vi "MoD Main-Optimize - HPLCv2 HWE.vi"() -> ()   [LabVIEW 2015]
uses:
  <vilib>/silver_ctls/ArrayMatrixCluster/Real Matrix NI_Silver.ctl
  <vilib>/ni845x/ni845x.llb/ni845xControl.ctl
  <vilib>/MakerHub/LINX/Public/Peripherals/Analog/Analog Read 1 Chan.vi
  <vilib>/MakerHub/LINX/Public/Peripherals/Analog/Analog Read N Chans.vi
  <vilib>/MakerHub/LINX/Public/Peripherals/Digital/Digital Write 1 Chan.vi
  <vilib>/MakerHub/LINX/Private/Local IO/LinxAnalogRead.vi
  <vilib>/MakerHub/LINX/Public/Utilities/Check Channel.vi
  <vilib>/MakerHub/LINX/Public/Peripherals/Digital/Digital Write N Chans.vi
  <vilib>/MakerHub/LINX/Private/Local IO/LinxDigitalWrite.vi
  <vilib>/addons/control/pid/pid.llb/PID Control Input Filter (DBL).vi
  <vilib>/MakerHub/LINX/Private/Utilties/Generate Error.vi
  <vilib>/addons/control/pid/autopid.llb/PID Online Autotuning (Relay Feedback).vi
  <vilib>/Analysis/Matrix/Numeric/Conversions/Array To Matrix - RA2.vi
  <vilib>/ni845x/ni845x.llb/NI-845x Close Device Reference.vi
  <vilib>/addons/control/pid/NI_PID_autopid.lvlib
  <vilib>/addons/control/pid/NI_PID_pid.lvlib
  <vilib>/Analysis/Matrix/NI_Matrix.lvlib
  <vilib>/MakerHub/LINX/LMH-LINX.lvlib
  <instrlib>/Harvard Apparatus PHD Ultra Series/Harvard Apparatus PHD Ultra Series.lvlib
panel:
  out "running?":bool=TRUE
  out "new_reactor_volume":bool[](array[boolean])
  out "new_reactor_length":bool[](array[boolean])
  out "Phase_Sensor_voltage":dbl
  out "P_tot":dbl
  out "pause for ms":bool=TRUE
  out "stop_xl_write":bool=TRUE
  out "Num_exp_till_pause":i32
  out "Syringe_pump?":bool=TRUE
  out "System Error":bool=TRUE
  out "error out":errorcluster
  out "Pump setpoint(ul/min) 6":dbl format="%#_13g"
  out "Pump setpoint(ul/min) 5":dbl format="%#_13g"
  out "Pump setpoint(ul/min) 4":dbl format="%#_13g"
  out "Pump setpoint(ul/min) 3":dbl format="%#_13g"
  out "Pump setpoint(ul/min) 2":dbl format="%#_13g"
  out "Pump setpoint(ul/min) 1":dbl format="%#_13g"
  out "Volume (ul) 5":dbl format="%#_13g"
  out "Volume (ul) 4":dbl format="%#_13g"
  out "Volume (ul) 3":dbl format="%#_13g"
  out "Volume (ul) 2":dbl format="%#_13g"
  out "Volume (ul) 1":dbl format="%#_13g"
  in  "tau 5":dbl format="%#_13g"
  out "tau 4":dbl format="%#_13g"
  out "tau 3":dbl format="%#_13g"
  out "tau 2":dbl format="%#_13g"
  out "tau 1":dbl format="%#_13g"
  out "Reactor Length":dbl format="%#_13g"
  out "Flowrate Sensor 2":dbl format="%#_13g"
  out "Flowrate Sensor 1":dbl format="%#_13g"
  out "Pressure 2":dbl format="%#_13g"
  out "Pressure 1":dbl format="%#_13g"
  out "Temperature Control 5":bool=TRUE
  out "Temperature Control 4":bool=TRUE
  out "Temperature Control 3":bool=TRUE
  out "Temperature Control 2":bool=TRUE
  out "Temperature Control 1":bool=TRUE
  out "Temperature SP 5":dbl format="%#_g'C"
  out "Temperature SP 4":dbl format="%#_g'C"
  out "Temperature SP 3":dbl format="%#_g'C"
  out "Temperature SP 2":dbl format="%#_g'C"
  out "Temperature SP 1":dbl format="%#_g'C"
  in  "Bay Temperature 5":dbl
  in  "SSR Duration 5":dbl
  in  "SSR Duration 4":dbl
  in  "SSR Duration 3":dbl
  in  "SSR Duration 2":dbl
  in  "SSR Duration 1":dbl
  in  "Total Product Amount":dbl=1.0 format="%#_gml"
  out "Setup Error":bool=TRUE
  out "Error Message":string
  out "ID CTR":i32
  in  "Tab Control":T1(tab)
  out "Reagent pic 5":picture
  in  "reagent name 5":string
  out "Reagent Pic 4":picture
  in  "reagent name 4":string
  out "Reagent Pic 3":picture
  in  "reagent  name 3":string="4-phenylcyclohexanone"
  in  "Product name":string
  in  "reagent name 1":string="Triethyl phosphonoacetate"
  out "Reagent Pic 1":picture
  in  "Vr5":dbl format="%#_guL"
  in  "Vr4":dbl format="%#_guL"
  in  "Vr3":dbl format="%#_guL"
  in  "Vr2":dbl format="%#_guL"
  in  "Vr1":dbl format="%#_guL"
  in  "System decide help Button":bool
  in  "Reaction Scheme Confirm":bool
  in  "Synthesis Route Array":string[][](array[string])=[["Triethyl phosphonoacetate", "0.2", "PhB(OH)2", "", "", ""], ["potassium tert-butoxide", "0.5", "-", "-", "-", "-"], ["4-phenylcyclohexanone", "0.2", "-", "-", "-", "-"], ["", "", "-", "-", "-", "-"]]
  in  "System decide help Button 2":bool
  out "Setup Confirm":bool=TRUE
  in  "BAY 1":u16(ring)=2 items=["               Bypass", "         Heated Reactor", "    Small Heated Reator", "         Cooled Reactor", "      Packed Bed Reactor", "          Photo Reactor", "             Separator"]
  in  "BAY 5":u16(ring) items=["               Bypass", "         Heated Reactor", "    Small Heated Reactor", "         Cooled Reactor", "     Packed Bed Reactor", "         Photo Reactor", "             Separator"]
  in  "BAY 4":u16(ring) items=["                Bypass", "         Heated Reactor", "    Small Heated Reactor", "         Cooled Reactor", "     Packed Bed Reactor", "         Photo Reactor", "             Separator"]
  in  "BAY 3":u16(ring) items=["               Bypass", "         Heated Reactor", "    Small Heated Reactor", "         Cooled Reactor", "     Packed Bed Reactor", "          Photo Reactor", "             Separator"]
  in  "BAY 2":u16(ring)=1 items=["               Bypass", "         Heated Reactor", "    Small Heated Reactor", "         Cooled Reactor", "      Packed Bed Reactor", "          Photo Reactor", "             Separator"]
  out "Reagent Pic 2":picture
  out "Product Pic":picture
  in  "reagent name 2":string="potassium tert-butoxide"
  in  "reagent name 6":string
  out "Reagent Pic 6":picture
  in  "System Parameters Help Button":bool
  out "Setup Confirm 2":bool
  in  "System Parameters Confirm Button":bool
  in  "Bay Parameters":T2={"Bay 1 "={"Pump 1 Flowrate"=0.0, "optimize_temp"=TRUE, "optimize_tau"=TRUE, "Run at set flowrate"=FALSE, "Pump 2 Flowrate"=0.0, "Temperature Params"=[40.0, 100.0, 100.0], "pump params 1"=[22.6, 226.0, 325.0], "pump params 2"=[22.6, 226.0, 325.0], "Temperature"=0.0, "Run at set temperature"=FALSE}, "Bay 2 "={"Pump 3 Flowrate"=0.0, "optimize_temp"=TRUE, "optimize_tau"=FALSE, "Run at set flowrate"=TRUE, "Temperature Params"=[40.0, 100.0, 100.0], "Resisdence time params"=[40.6, 406.0, 650.0], "pump_at_ratio"=FALSE, "pump_num_ratio"=1.0, "Temperature"=0.0, "Run at set temperature"=FALSE}, "Bay 3 "={"Pump 4 Flowrate"=100.0, "optimize_temp"=FALSE, "optimize_tau"=FALSE, "Run at set flowrate"=FALSE, "Temperature Params"=[40.0, 100.0, 100.0], "Resisdence time params"=[47.0, 476.0, 0.0], "pump_at_ratio"=FALSE, "pump_num_ratio"=0.0, "Temperature "=0.0, "Run at set temperature"=FALSE}, "Bay 4 "={"Pump 5 Flowrate"=40.0, "Run at set flowrate"=FALSE, "optimize_temp"=FALSE, "optimize_tau"=TRUE, "Resisdence time params"=[40.6, 406.0, 225.0], "Temperature Params"=[40.0, 100.0, 80.0], "pump_at_ratio"=FALSE, "pump_num_ratio"=0.0, "Temperature"=0.0, "Run at set temperature"=FALSE}, "Bay 5 "={"Pump 6 Flowrate"=0.0, "Run at set flowrate"=FALSE, "optimize_temp"=FALSE, "optimize_tau"=FALSE, "Resisdence time params"=[0.0, 0.0, 0.0], "Temperature Params"=[0.0, 0.0, 0.0], "pump_at_ratio"=FALSE, "pump_num_ratio"=0.2, "Temperature"=0.0, "Run at set temperature"=FALSE}, "Excel File Name"="C:\\Users\\HPLC\\Dropbox (MIT)\\MoD Files\\Data\\HWE_050517c", "hplc File Name"="C:\\Chem32\\1\\Data\\MOD", "Matlab File"="C:\\Users\\HPLC\\Dropbox (MIT)\\MoD Files\\Data\\HWE_051017_2", "Syringe for Pump 2?"=FALSE, "Num_conditons_per_wait"=1.0, "Continue from previous optimization?"=FALSE, "Total Number of Experiments 2"=33.0, "Hplc Wait time(min)"=6.0, "increas_decrease_hplc_peak"=FALSE, "Internal Standard?"=TRUE, "ISTD start"=2.5, "ISTD end"=3.4, "hplc_start"=3.5, "hplc_end"=6.0, "throughput_yield"=TRUE} {"Hplc Wait time(min)" format="%#_13g"; "Bay 5"."Temperature Params" format="%#_g'C"; "Bay 4"."Temperature Params" format="%#_g'C"; "Bay 3"."Temperature Params" format="%#_g'C"; "Bay 2"."Temperature Params" format="%#_g'C"; "Bay 1"."Temperature Params" format="%#_g'C"}
  out "System Confirm Not Clicked":string
  out "best_exp_num":dbl=1.0
  out "temperature_best":dbl[](array[numeric])
  out "Flowrates(ul/min)_best":dbl[](array[numeric])
  out "System Status":u16(ring)=2 caption="Sy" items=["System  Error", "System Running", "System Standby"]
  out "Current Experiment":dbl=1.0
  out "Total Number of Experiments":dbl=33.0
  out "Phase Sensor Chart":T3(graph)
  out "HPLC Analysis":bool
  out "Equlibrating Temperature":bool
  out "Flushing System":bool
  out "Calculate condition":bool
  out "Temperature 5":dbl format="%#_g'C"
  out "Temperature 4":dbl format="%#_g'C"
  out "Temperature 3":dbl format="%#_g'C"
  out "Temperature 2":dbl format="%#_g'C"
  out "Temperature 1":dbl format="%#_g'C"
  out "Flowrate Chart":T4(graph)
  out "Teperature Chart":T3(graph)
  out "Pump Setpoints Chart":T3(graph)
  out "Pressure Chart":T3(graph)
  out "Optimization_loop_index":i32
  out "curr_wait_time":dbl
  out "total_flush_time":dbl
  out "Temp SS? 5":bool=TRUE
  out "Temp SS? 4":bool=TRUE
  out "Temp SS? 3":bool=TRUE
  out "Temp SS? 2":bool=TRUE
  out "Temp SS? 1":bool=TRUE
  out "System Flushed?":bool
  out "stop_button clicked":bool
  out "experiment history":T5
  in  "Number of System Flushes per condtion":dbl=2.5
  in  "calculate volume 3":bool
  in  "calculate volume 2":bool=TRUE
  in  "calculate volume 1":bool=TRUE
  in  "calculate volume 4":bool
  in  "calculate volume 5":bool
  in  "Extra system dead volume":dbl format="%#_gul"
  in  "new reactor length? 1":bool
  in  "tube_length(in)":dbl[](array[numeric])=[188.0, 188.0, 10.0, 10.0, 10.0]
  out "Pause Before Analysis":bool
  out "Chiller COMM Port":bool
  out "Arduino COMM Port 2":bool
  out "Temperature Sensor COMM Port":bool
  out "Flow Rate":bool
  out "Pressure":bool
  out "Pump COMM Port":bool
  in  "COMM Port :: Milligat Pumps":refnum<visa-resource-name>="COM10"
  in  "Arduino COMM Port":refnum<visa-resource-name>="COM3"
  in  "Sample Valve COMM::Port":refnum<visa-resource-name>="COM6"
  in  "COMM Port:: Harvard Syringe Pump":refnum<visa-resource-name>="COM5"
  in  "tube_id(in)":enum16{".01", ".02", ".03", ".04"}[](array[ring])=[enum.".03", enum.".03", enum.".03", enum.".03", enum.".03"]
  out "Total System Resisdence Time(min)":dbl
  in  "Debug_run_button":bool
  in  "new reactor length? 2":bool
  in  "new reactor length? 3":bool
  in  "new reactor length? 4":bool
  in  "new reactor length? 5":bool
  in  "IR Sensor Device":T6="USB0::0x3923::0x7514::01B3FF21::RAW"
  out "Stop":bool=TRUE
  in  "Run_Stop_cluster":T7
  # "Molecules on Demand"
  # "Synthetic Route"
  # "5"
  # "6"
  # "4"
  # "Product"
  # "1"
  # "2"
  # "3"
  # "Reagent List"
  # "Concentration(M)"
  # "Molecule"
  # "1"
  # "1"
  # "2"
  # "2"
  # "3"
  # "3"
  # "4"
  # "4"
  # "5"
  # "6"
  # "5"
  # "6"
  # "Product"
  # "Reactor Volume:"
  # "Optimization Parameters"
  # "Pause after"
  # "Experiments"
  # "Optimize for"
  # "to"
  # "of HPLC Peak from"
  # "from"
  # "to"
  # "min"
  # "min"
  # "HPLC runtime"
  # "# Iterations"
  # "Reporting"
  # "Excel Output File Name"
  # "HPLC File Path"
  # "MATLAB File Path"
  # "Temperature"
  # "Flowrate(ul/min)"
  # "Lower Bound"
  # "Upper Bound"
  # "Optimize?"
  # "-or-"
  # "Run at"
  # "times incoming flow"
  # "Setpoint"
  # "Temperature"
  # "Flowrate(ul/min)"
  # "Lower Bound"
  # "Upper Bound"
  # "Optimize?"
  # "-or-"
  # "Run at"
  # "times incoming flow"
  # "Setpoint"
  # "Temperature"
  # "Flowrate(ul/min)"
  # "Lower Bound"
  # "Upper Bound"
  # "Optimize?"
  # "-or-"
  # "Run at"
  # "times incoming flow"
  # "Setpoint"
  # "Temperature"
  # "Flowrate 3 (ul/min)"
  # "Lower Bound"
  # "Upper Bound"
  # "Optimize?"
  # "-or-"
  # "Run at"
  # "times incoming flow"
  # "Setpoint"
  # "Temperature"
  # "Flowrate 1(ul/min)"
  # "Flowrate 2(ul/min)"
  # "Lower Bound"
  # "Upper Bound"
  # "Optimize?"
  # "Setpoint"
  # "Pressure (psi)"
  # "System Status"
  # "Temperature('C)"
  # "BAY"
  # "1"
  # "2"
  # "3"
  # "4"
  # "5"
  # "Pump Flowrate Setpoint(ul/min)"
  # "Flowrate (ul/min)"
  # "Phase Sensor"
  # "Current Experiment"
  # "Temperature('C)"
  # "Flowrate(ul/min)"
  # "Exp"
  # "Current Best Condition"
  # "Time to reach steady state:"
  # "Current Wait Time:"
  # "Experimental Steps"
  # "Calculated New Conditions"
  # "Steady State"
  # "Analyzed HPLC"
  # "Equilibrated Temperature"
  # "Tube Length (cm)"
  # "Bay"
  # "Tube ID (in)"
  # "Calculate Volume"
  # "Use new tube length"
  # "1."
  # "2."
  # "3."
  # "4."
  # "5."
  # "Reactor Lengths\n*Heated Reactor - 188cm * Small Reactor - 99cm * Bypass - 10cm * Separator - *"
  # "All Experimental Data"
  # "P1"
  # "P2"
  # "P3"
  # "P4"
  # "P5"
  # "P6"
  # "T1"
  # "T2"
  # "T3"
  # "T4"
  # "T5"
  # "Obj_fun"
  # "HPLC_Data"
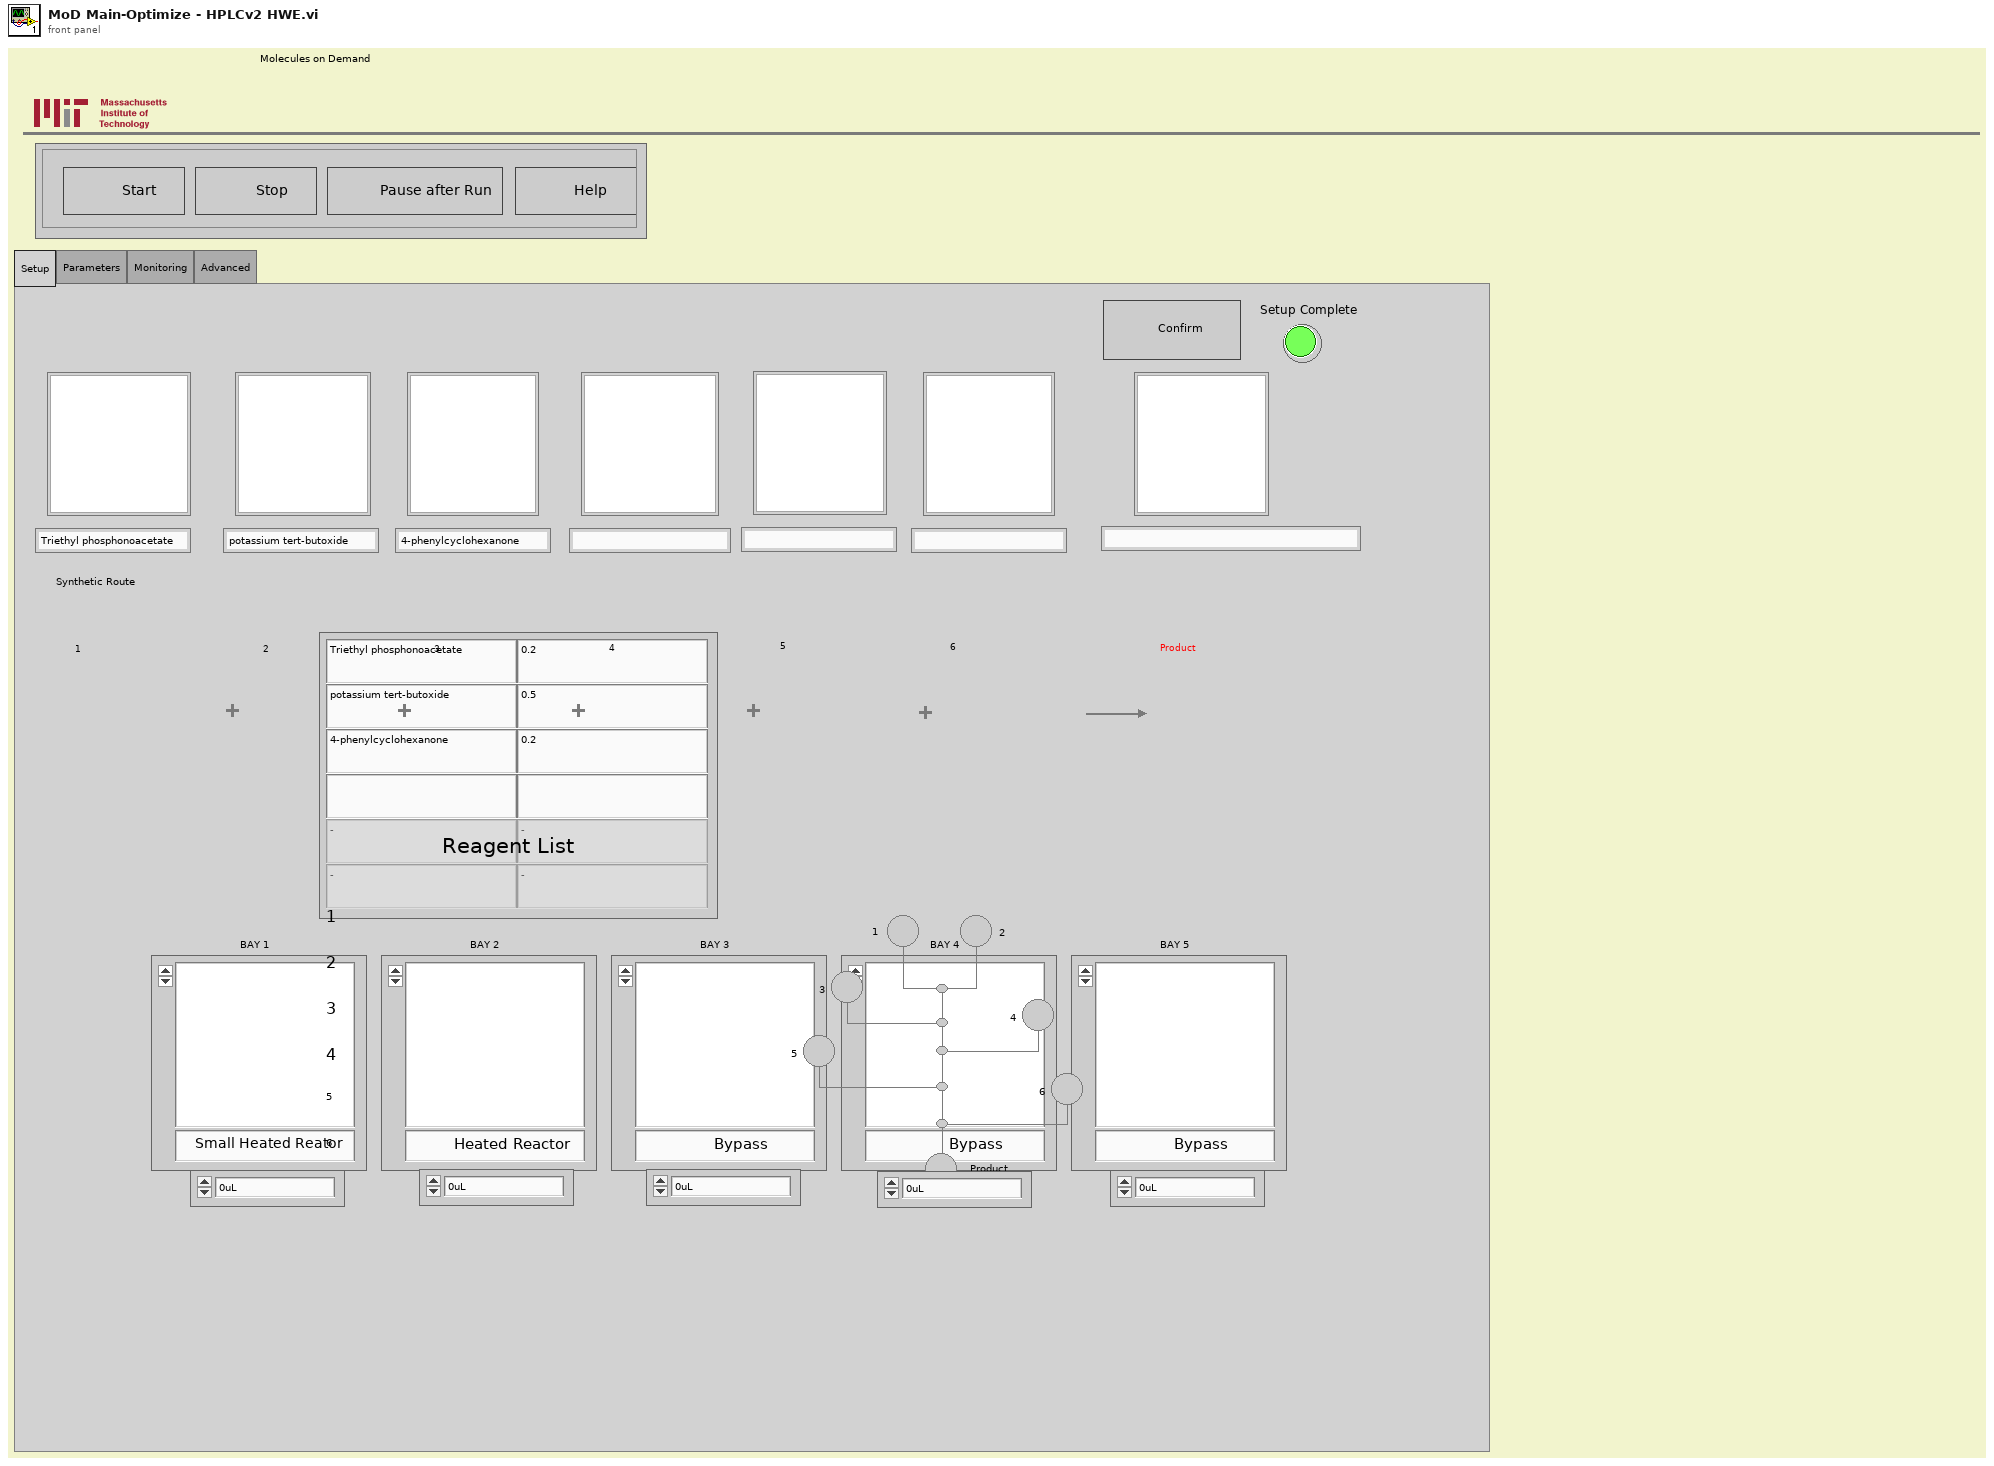
[diagram p1: front panel]
types:
  T1 = enum32{"Setup", "Parameters", "Monitoring", "Advanced"}
  T2 = cluster{"Bay 1 ":cluster{"Pump 1 Flowrate":dbl, "optimize_temp":bool, "optimize_tau":bool, "Run at set flowrate":bool, "Pump 2 Flowrate":dbl, "Temperature Params":dbl[], "pump params 1":dbl[], "pump params 2":dbl[], "Temperature":dbl, "Run at set temperature":bool}, "Bay 2 ":cluster{"Pump 3 Flowrate":dbl, "optimize_temp":bool, "optimize_tau":bool, "Run at set flowrate":bool, "Temperature Params":dbl[], "Resisdence time params":dbl[], "pump_at_ratio":bool, "pump_num_ratio":dbl, "Temperature":dbl, "Run at set temperature":bool}, "Bay 3 ":cluster{"Pump 4 Flowrate":dbl, "optimize_temp":bool, "optimize_tau":bool, "Run at set flowrate":bool, "Temperature Params":dbl[], "Resisdence time params":dbl[], "pump_at_ratio":bool, "pump_num_ratio":dbl, "Temperature ":dbl, "Run at set temperature":bool}, "Bay 4 ":cluster{"Pump 5 Flowrate":dbl, "Run at set flowrate":bool, "optimize_temp":bool, "optimize_tau":bool, "Resisdence time params":dbl[], "Temperature Params":dbl[], "pump_at_ratio":bool, "pump_num_ratio":dbl, "Temperature":dbl, "Run at set temperature":bool}, "Bay 5 ":cluster{"Pump 6 Flowrate":dbl, "Run at set flowrate":bool, "optimize_temp":bool, "optimize_tau":bool, "Resisdence time params":dbl[], "Temperature Params":dbl[], "pump_at_ratio":bool, "pump_num_ratio":dbl, "Temperature":dbl, "Run at set temperature":bool}, "Excel File Name":string, "hplc File Name":string, "Matlab File":string, "Syringe for Pump 2?":bool, "Num_conditons_per_wait":dbl, "Continue from previous optimization?":bool, "Total Number of Experiments 2":dbl, "Hplc Wait time(min)":dbl, "increas_decrease_hplc_peak":bool, "Internal Standard?":bool, "ISTD start":dbl, "ISTD end":dbl, "hplc_start":dbl, "hplc_end":dbl, "throughput_yield":bool}
  T3 = cluster{"[0]":dbl, "[1]":dbl, "[2]":dbl, "[3]":dbl, "[4]":dbl, "[5]":dbl, "[6]":dbl, "[7]":dbl, "[8]":dbl}
  T4 = cluster{"[0]":i32, "[1]":i32, "[2]":i32, "[3]":i32, "[4]":i32, "[5]":i32, "[6]":i32, "[7]":i32, "[8]":i32}
  T5 = typedef "Real Matrix NI_Silver.ctl" = dbl[][]
  T6 = typedef "ni845xControl.ctl" = refnum<k21>
  T7 = cluster{"Stop":bool, "Run":bool, "Stop Run Button":bool, "Help Button":bool}
  T8 = cluster{"Proportional gain Kc":dbl, "Integral time Ti (sec)":dbl, "Derivative time Ti (sec)":dbl}
  T9 = cluster{"type of controller":enum16{"P", "PI", "PID"}, "relay cycles":i32, "relay amplitude":dbl, "control specifications":enum16{"Fast", "Normal", "Slow"}, "PV noise level":dbl}
  T10 = typedef "LMH-LINX.lvlib/LINX Ref.ctl" = cluster{"IO":T11, "Interface":T12, "LINX Device Config":T13}
  T11 = typedef "LMH-LINX.lvlib/Platform.ctl" = enum16{"Remote", "Local"}
  T12 = typedef "LMH-LINX.lvlib/Interface.ctl" = enum16{"Serial", "TCP"}
  T13 = typedef "LMH-LINX.lvlib/Device.lvlib/LINX Device Config.ctl" = cluster{"Interface":T12, "COM Port":refnum<visa-resource-name>, "TCP Configuration":T14, "Device Family":u8, "Device ID":u8, "Device Name":string, "TCP Ref":refnum<k5>, "Channels":T15}
  T14 = typedef "LMH-LINX.lvlib/Device.lvlib/TCP Config.ctl" = cluster{"IP Address":string, "Port":u16}
  T15 = typedef "LMH-LINX.lvlib/Channels.ctl" = cluster{"DI":u8[], "DO":u8[], "AI":u8[], "AO":u8[], "PWM":u8[], "QE":u8[], "UART":u8[], "I2C 2":u8[], "SPI":u8[], "CAN":u8[], "Servo":u8[], "AI Ref (V)":dbl, "AI Resolution (Bits)":u8, "AO Ref (V)":dbl, "AO Resolution (Bits)":u8}
  T16 = typedef "imagedata.ctl" = cluster{"image type":i32, "image depth":i32, "image":u8[], "mask":u8[], "colors":u32[], "Rectangle":cluster{"left":i16, "top":i16, "right":i16, "bottom":i16}}
  T17 = cluster{"proportional gain (Kc)":dbl, "integral time (Ti, min)":dbl, "derivative time (Td, min)":dbl}
  T18 = typedef "NI_Matrix.lvlib/RealMatrix.ctl" = dbl[][]
  T19 = enum16{"Left Button", "Center Button", "Right Button", "Window Close"}
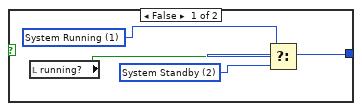
[diagram p3: hidden frame]
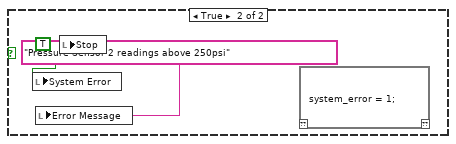
[diagram p4: hidden frame]
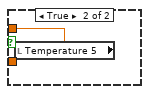
[diagram p6: hidden frame]
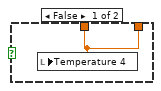
[diagram p7: hidden frame]
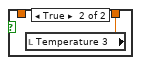
[diagram p8: hidden frame]
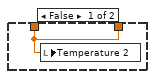
[diagram p9: hidden frame]
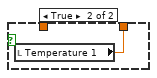
[diagram p10: hidden frame]
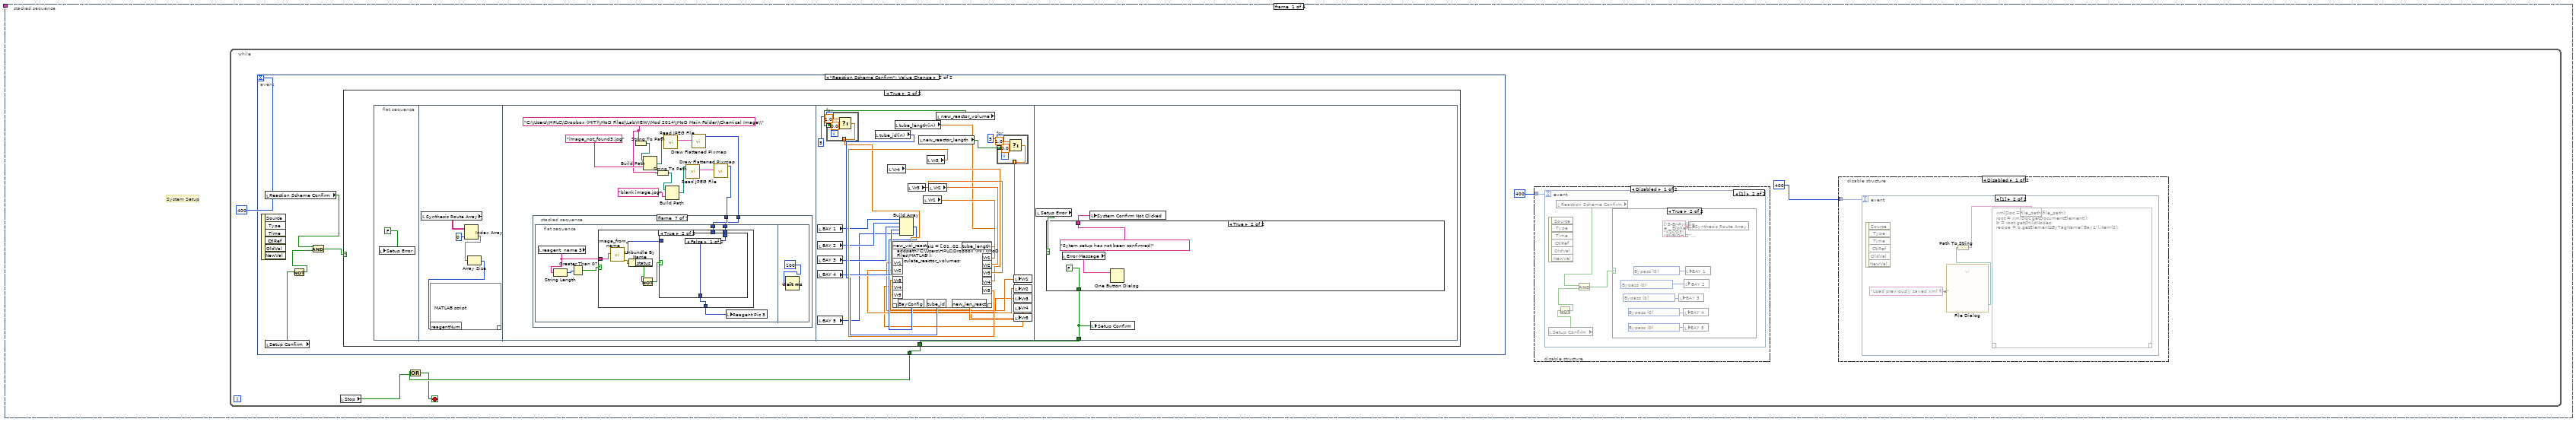
[diagram p11: hidden frame]
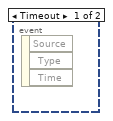
[diagram p12: hidden frame]
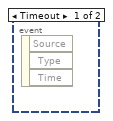
[diagram p14: hidden frame]
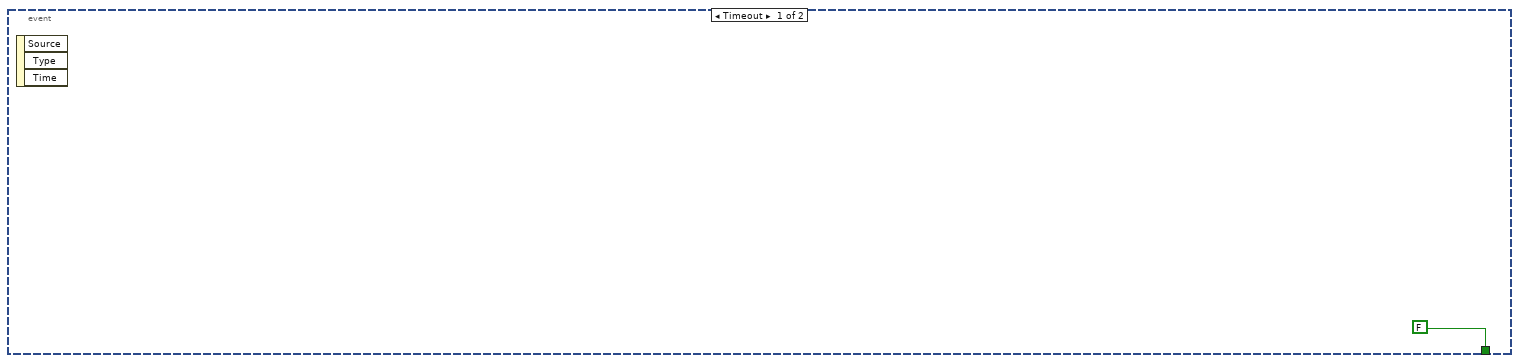
[diagram p17: hidden frame]
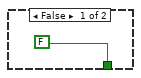
[diagram p18: hidden frame]
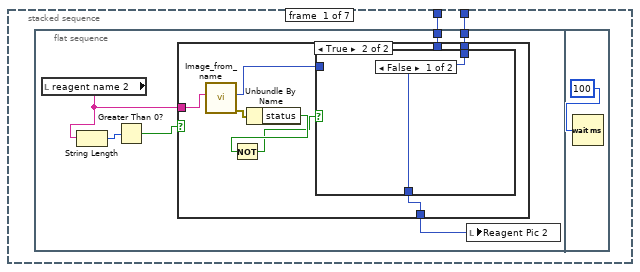
[diagram p19: hidden frame]
diagram:
  # "Assume User always uses the first bay first"
  n1 = flat-sequence {
    tunnel: ["COMM Port :: Milligat Pumps"] -> w9
    tunnel: ["Arduino COMM Port"] -> w8
    tunnel: [w11] -> w5
    tunnel: ["Bay Parameters"] -> w4
    tunnel: [w60] -> w10
    tunnel: w9 -> [w60]
    tunnel: w8 -> [w48]
    tunnel: [w54] -> w7
    tunnel: [w52] -> w6
    tunnel: w5 -> [w52]
    tunnel: w4 -> [w50]
    tunnel: [w47] -> w3
    tunnel: w10 -> [w66]
    tunnel: w7 -> [w65]
    tunnel: w6 -> [w63]
    tunnel: w3 -> [w61]
    tunnel: [w61] -> w1
    tunnel: [w1345] -> w2
    tunnel: w1 -> [w1345]
    tunnel: w2 -> [w1346]
    frame #0 {
      w36 = FALSE ("Equlibrating Temperature")
      n2 = script code="TempArr1=[23 23 23 23 23 23 23 23 23 23]';\nTempArr2=[23 23 23 23 23 23 23 23 23 23]';\nTempArr3=[23 23 23 23 23 23 23 23 23 23]';\nTempArr4=[23 23 23 23 23 23 23 23 23 23]';\nTempArr5=[23 23 23 23 23 23 23 23 23 23]';\ntemp_error1 =0;\ntemp_error2 =0;\ntemp_error3 =0;\ntemp_error4 =0;\ntemp_error5 =0;\ntemp_check1 = 0;\ntemp_check2 = 0;\ntemp_check3 = 0;\ntemp_check4 = 0;\ntemp_check5 = 0;\nT1=23;\nT2=23;\nT3=23;\nT4=23;\nT5=23;"() -> ()  [unwired: 1 in, 1 out]
      n3 = Build Array("calculate volume 1", "calculate volume 2", "calculate volume 3", "calculate volume 4", "calculate volume 5") -> (→"new_reactor_volume":bool[])
      n4 = Build Array("new reactor length? 1", "new reactor length? 2", "new reactor length? 3", "new reactor length? 4", "new reactor length? 5") -> (→"new_reactor_length":bool[])
      n5 = call <vilib>:"Initialize.vi"("VISA resource name"="COMM Port:: Harvard Syringe Pump") -> ("VISA resource name out"=w11:refnum<visa-resource-name>)  [unwired: 9 in, 1 out]
      "Stop" <- FALSE ("Stop")
      "ID CTR" <- 0
      "Setup Confirm" <- FALSE ("Setup Confirm")
      "Error Message" <- "System shutdown sucessfully. No errors to report." ("Error Message")
      "Setup Error" <- FALSE ("Setup Error")
      "Reactor Length" <- 10.5
      "System Error" <- FALSE ("System Error")
      "Num_exp_till_pause" <- 0 ("Num_exp_till_pause")
      "Equlibrating Temperature" <- w36
      "Calculate condition" <- w36
      "Flushing System" <- w36
      "HPLC Analysis" <- w36
      "stop_xl_write" <- FALSE ("stop_xl_write")
      "Pump setpoint(ul/min) 1" <- 0.0 ("Pump setpoint(ul/min) 1")
      "Pump setpoint(ul/min) 2" <- 0.0 ("Pump setpoint(ul/min) 2")
      "Pump setpoint(ul/min) 4" <- 0.0 ("Pump setpoint(ul/min) 4")
      "Pump setpoint(ul/min) 6" <- 0.0 ("Pump setpoint(ul/min) 6")
      "Pump setpoint(ul/min) 3" <- 0.0 ("Pump setpoint(ul/min) 3")
      "Pump setpoint(ul/min) 5" <- 0.0 ("Pump setpoint(ul/min) 5")
      "pause for ms" <- FALSE ("pause for ms")
      "Setup Confirm 2" <- FALSE ("Setup Confirm 2")
      "running?" <- FALSE ("running?")
    }
    frame #1 {
      w49 = FALSE
      w59 = 23
      (unwired) path "C:/Users/User1/Documents/Lab/MoD/Images"
      n6 = disable-structure shown="Disabled" {
        frame Disabled {
          n7 = local read "BAY 2"() -> ()  [unwired: 1 out]
          n8 = local read "BAY 3"() -> ()  [unwired: 1 out]
          n9 = local read "BAY 4"() -> ()  [unwired: 1 out]
          n10 = local read "BAY 5"() -> ()  [unwired: 1 out]
          n11 = local read "BAY 1"() -> ()  [unwired: 1 out]
        }
        frame Enabled {
        }
      }
      n12 = local write "Debug_run_button"(TRUE) -> ()
      n13 = call <vilib>:"Initialize.vi"("Serial Port"=w48) -> ("LINX Resource"=w47:T10)  [unwired: 8 in, 2 out]
      n14 = local write "System Parameters Confirm Button"(w49) -> ()
      n15 = local write "Setup Confirm 2"(w49) -> ()
      n16 = Unbundle By Name(w50) -> ("Syringe for Pump 2?"=→"Syringe_pump?":bool)
      n17 = local write "Temperature 1"(w59) -> ()
      n18 = local write "Temperature 2"(w59) -> ()
      n19 = local write "Temperature 3"(w59) -> ()
      n20 = local write "Temperature 4"(w59) -> ()
      n21 = local write "Temperature 5"(w59) -> ()
      n22 = local write "Temperature SP 1"(w59) -> ()
      n23 = local write "Temperature SP 2"(w59) -> ()
      n24 = local write "Temperature SP 3"(w59) -> ()
      n25 = local write "Temperature SP 4"(w59) -> ()
      n26 = local write "Temperature SP 5"(w59) -> ()
      n27 = Current VI's Path() -> (path=w58:path)
      n28 = Strip Path(path=w58) -> (stripped path=w56:path)  [unwired: 1 out]
      n29 = Strip Path(path=w56) -> (stripped path=w55:path)  [unwired: 1 out]
      n30 = Build Path(base path=w55, name or relative path="MATLAB") -> (appended path=w54:path)
    }
    frame #2 {
      # "Main Help Dialog Popup"
      n31 = while {
        stop <- w1339 stop-if-true
        n32 = event shown="[6] \"Run_Stop_cluster.Run\": Value Change" {
          selector: _ -> [_ _ _ _ _ _ _]
          dyn-events: _ -> [_ _ _ _ _ _ _]
          timeout: 100 -> [_ _ _ _ _ _ _]
          event Timeout {
            n33 = event-data() -> ()  [unwired: 1 in, 3 out]
          }
          event "Run_Stop_cluster.Help Button": Value Change {
            n34 = local read "Run_Stop_cluster"() -> (w1342:T7)
            n35 = event-data() -> ()  [unwired: 1 in, 4 out]
            n36 = Unbundle By Name(w1342) -> ("Help Button"=w1341:bool)
            n37 = case shown="True" w1341 {
              frame False {
              }
              frame True {
                n38 = call "help.vi"() -> ()  [unwired: 11 in]
              }
            }
          }
          event "System decide help Button": Value Change {
            n39 = event-data() -> ()  [unwired: 1 in, 5 out]
            n40 = call "help_synthesis_man-auto_instructions.vi"() -> ()  [unwired: 12 in]
          }
          event "System Parameters Help Button": Value Change {
            n41 = event-data() -> ()  [unwired: 1 in, 5 out]
            n42 = call "help_parameters_setup.vi"() -> ()  [unwired: 12 in]
          }
          event "System decide help Button 2": Value Change {
            n43 = event-data() -> ()  [unwired: 1 in, 5 out]
            n44 = call "help_synthesis_route_instructions.vi"() -> ()  [unwired: 12 in]
          }
          event "Run_Stop_cluster.Stop": Value Change {
            n45 = event-data() -> ()  [unwired: 1 in, 5 out]
            n46 = local write "Stop"(TRUE) -> ()
          }
          event "Run_Stop_cluster.Run": Value Change {
            n47 = event-data() -> ()  [unwired: 1 in, 5 out]
            n48 = local write "running?"(TRUE) -> ()
          }
        }
        n49 = local read "Stop"() -> (w1339:bool)
      }
      n50 = stacked-sequence {
        tunnel: w66 -> [_ _ _ _]
        tunnel: w65 -> [_ w425 _ _]
        tunnel: w63 -> [_ _ _ w592]
        tunnel: w61 -> [_ _ _ w590]
        frame #0 {
          # "System Setup"
          n51 = while {
            stop <- w200 stop-if-true
            n52 = event shown="[1] \"Reaction Scheme Confirm\": Value Change" {
              selector: _ -> [_ _]
              dyn-events: _ -> [_ _]
              timeout: 400 -> [_ _]
              tunnel: [FALSE w220] -> w202
              event Timeout {
                n53 = event-data() -> ()  [unwired: 1 in, 3 out]
              }
              event "Reaction Scheme Confirm": Value Change {
                n54 = event-data() -> ()  [unwired: 1 in, 6 out]
                n55 = local read "Reaction Scheme Confirm"() -> (w224:bool)
                n56 = local read "Setup Confirm"() -> (w222:bool)
                n57 = Not(x=w222) -> (.not. x?=w221:bool)
                n58 = And(x=w224, y=w221) -> (x .and. y?=w223:bool)
                n59 = case shown="True" w223 {
                  tunnel: [FALSE w226] -> w220
                  frame False {
                  }
                  frame True {
                    n60 = flat-sequence {
                      tunnel: [w415] -> w226
                      frame #0 {
                        n61 = local write "Setup Error"(FALSE) -> ()
                      }
                      frame #1 {
                        n62 = local read "Synthesis Route Array"() -> (w230:string[][])
                        n63 = Index Array(array=w230, index (col)=0 ("disabled index (col)")) -> (element=w228:string[])  [unwired: 1 in]
                        n64 = Array Size(array=w228) -> (size(s)=w231:i32)
                        n65 = script code="MATLAB script"("reagentNum"=w231) -> ()  [unwired: 1 in, 1 out]
                      }
                      frame #2 {
                        w234 = "C:\\Users\\HPLC\\Dropbox (MIT)\\MoD Files\\LabVIEW\\Mod 2014\\MoD Main Folder\\Chemical Image\\" ("string")
                        n66 = String To Path(string=w234) -> (path=w240:path)
                        n67 = Build Path(base path=w240, name or relative path="image_not_found3.jpg") -> (appended path=w239:path)
                        n68 = String To Path(string=w234) -> (path=w237:path)
                        n69 = call <vilib>:"Read JPEG File.vi"("path to JPEG file"=w239) -> ("image data"=w242:T16)  [unwired: 1 in, 9 out]
                        n70 = Build Path(base path=w237, name or relative path="blank image.jpg") -> (appended path=w235:path)
                        n71 = call <vilib>:"Read JPEG File.vi"("path to JPEG file"=w235) -> ("image data"=w238:T16)  [unwired: 1 in, 9 out]
                        n72 = call <vilib>:"Draw Flattened Pixmap.vi"("image data"=w242) -> ("new picture"=w233:picture)  [unwired: 3 in, 5 out]
                        n73 = call <vilib>:"Draw Flattened Pixmap.vi"("image data"=w238) -> ("new picture"=w232:picture)  [unwired: 3 in, 5 out]
                        n74 = stacked-sequence {
                          tunnel: w233 -> [w244 w264 w284 w304 w324 w343 w363]
                          tunnel: w232 -> [w243 w263 w283 w303 w323 w344 w364]
                          frame #0 {
                            n75 = flat-sequence {
                              tunnel: w244 -> [w250]
                              tunnel: w243 -> [w248]
                              frame #0 {
                                n76 = local read "reagent name 2"() -> (w246:string)
                                n77 = String Length(string=w246) -> (length=w249:i32)
                                n78 = Greater Than 0?(x=w249) -> (x > 0?=w247:bool)
                                n79 = case shown="True" w247 {
                                tunnel: w250 -> [_ w256]
                                tunnel: w248 -> [w251 _]
                                tunnel: [w251 w255] -> w245
                                tunnel: w246 -> [_ w254]
                                frame False {
                                }
                                frame True {
                                n80 = call "Image_from_name.vi"("Chemical Name"=w254) -> ("error out"=w257:errorcluster, "Downloaded Picture"=w258:picture)  [unwired: 8 in, 1 out]
                                n81 = Unbundle By Name(w257) -> ("status"=w253:bool)
                                n82 = Not(x=w253) -> (.not. x?=w252:bool)
                                n83 = case shown="False" w252 {
                                tunnel: w258 -> [_ w261]
                                tunnel: [w259 w260] -> w255
                                tunnel: w256 -> [w259 _]
                                frame False {
                                }
                                frame True {
                                n84 = call <vilib>:"Draw Flattened Pixmap.vi"("picture"=w261) -> ("new picture"=w260:picture)  [unwired: 8 in]
                                }
                                }
                                }
                                }
                                n85 = local write "Reagent Pic 2"(w245) -> ()
                              }
                              frame #1 {
                                n86 = Wait (ms)(milliseconds to wait=100) -> ()  [unwired: 1 out]
                              }
                            }
                          }
                          frame #1 {
                            n87 = flat-sequence {
                              tunnel: w264 -> [w270]
                              tunnel: w263 -> [w268]
                              frame #0 {
                                n88 = local read "reagent name 1"() -> (w265:string)
                                n89 = String Length(string=w265) -> (length=w269:i32)
                                n90 = Greater Than 0?(x=w269) -> (x > 0?=w267:bool)
                                n91 = case shown="True" w267 {
                                tunnel: w270 -> [_ w276]
                                tunnel: w268 -> [w271 _]
                                tunnel: [w271 w275] -> w266
                                tunnel: w265 -> [_ w274]
                                frame False {
                                }
                                frame True {
                                n92 = call "Image_from_name.vi"("Chemical Name"=w274) -> ("error out"=w277:errorcluster, "Downloaded Picture"=w278:picture)  [unwired: 8 in, 1 out]
                                n93 = Unbundle By Name(w277) -> ("status"=w273:bool)
                                n94 = Not(x=w273) -> (.not. x?=w272:bool)
                                n95 = case shown="True" w272 {
                                tunnel: w278 -> [_ w281]
                                tunnel: [w279 w280] -> w275
                                tunnel: w276 -> [w279 _]
                                frame False {
                                }
                                frame True {
                                n96 = call <vilib>:"Draw Flattened Pixmap.vi"("picture"=w281) -> ("new picture"=w280:picture)  [unwired: 8 in]
                                }
                                }
                                }
                                }
                                n97 = local write "Reagent Pic 1"(w266) -> ()
                              }
                              frame #1 {
                                n98 = Wait (ms)(milliseconds to wait=100) -> ()  [unwired: 1 out]
                              }
                            }
                          }
                          frame #2 {
                            n99 = flat-sequence {
                              tunnel: w284 -> [w290]
                              tunnel: w283 -> [w288]
                              frame #0 {
                                n100 = local read "Product name"() -> (w285:string)
                                n101 = String Length(string=w285) -> (length=w289:i32)
                                n102 = Greater Than 0?(x=w289) -> (x > 0?=w287:bool)
                                n103 = case shown="True" w287 {
                                tunnel: w290 -> [_ w296]
                                tunnel: w288 -> [w291 _]
                                tunnel: [w291 w295] -> w286
                                tunnel: w285 -> [_ w294]
                                frame False {
                                }
                                frame True {
                                n104 = call "Image_from_name.vi"("Chemical Name"=w294) -> ("error out"=w297:errorcluster, "Downloaded Picture"=w298:picture)  [unwired: 8 in, 1 out]
                                n105 = Unbundle By Name(w297) -> ("status"=w292:bool)
                                n106 = Not(x=w292) -> (.not. x?=w293:bool)
                                n107 = case shown="False" w293 {
                                tunnel: w298 -> [_ w301]
                                tunnel: [w299 w300] -> w295
                                tunnel: w296 -> [w299 _]
                                frame False {
                                }
                                frame True {
                                n108 = call <vilib>:"Draw Flattened Pixmap.vi"("picture"=w301) -> ("new picture"=w300:picture)  [unwired: 8 in]
                                }
                                }
                                }
                                }
                                n109 = local write "Product Pic"(w286) -> ()
                              }
                              frame #1 {
                                n110 = Wait (ms)(milliseconds to wait=100) -> ()  [unwired: 1 out]
                              }
                            }
                          }
                          frame #3 {
                            n111 = flat-sequence {
                              tunnel: w304 -> [w310]
                              tunnel: w303 -> [w308]
                              frame #0 {
                                n112 = local read "reagent name 6"() -> (w305:string)
                                n113 = String Length(string=w305) -> (length=w309:i32)
                                n114 = Greater Than 0?(x=w309) -> (x > 0?=w307:bool)
                                n115 = case shown="True" w307 {
                                tunnel: w310 -> [_ w316]
                                tunnel: w308 -> [w311 _]
                                tunnel: [w311 w315] -> w306
                                tunnel: w305 -> [_ w314]
                                frame False {
                                }
                                frame True {
                                n116 = call "Image_from_name.vi"("Chemical Name"=w314) -> ("error out"=w317:errorcluster, "Downloaded Picture"=w318:picture)  [unwired: 8 in, 1 out]
                                n117 = Unbundle By Name(w317) -> ("status"=w312:bool)
                                n118 = Not(x=w312) -> (.not. x?=w313:bool)
                                n119 = case shown="False" w313 {
                                tunnel: w318 -> [_ w321]
                                tunnel: [w319 w320] -> w315
                                tunnel: w316 -> [w319 _]
                                frame False {
                                }
                                frame True {
                                n120 = call <vilib>:"Draw Flattened Pixmap.vi"("picture"=w321) -> ("new picture"=w320:picture)  [unwired: 8 in]
                                }
                                }
                                }
                                }
                                n121 = local write "Reagent Pic 6"(w306) -> ()
                              }
                              frame #1 {
                                n122 = Wait (ms)(milliseconds to wait=100) -> ()  [unwired: 1 out]
                              }
                            }
                          }
                          frame #4 {
                            n123 = flat-sequence {
                              tunnel: w324 -> [w330]
                              tunnel: w323 -> [w328]
                              frame #0 {
                                n124 = local read "reagent name 5"() -> (w325:string)
                                n125 = String Length(string=w325) -> (length=w329:i32)
                                n126 = Greater Than 0?(x=w329) -> (x > 0?=w327:bool)
                                n127 = case shown="True" w327 {
                                tunnel: w330 -> [_ w336]
                                tunnel: w328 -> [w331 _]
                                tunnel: [w331 w335] -> w326
                                tunnel: w325 -> [_ w334]
                                frame False {
                                }
                                frame True {
                                n128 = call "Image_from_name.vi"("Chemical Name"=w334) -> ("error out"=w337:errorcluster, "Downloaded Picture"=w338:picture)  [unwired: 8 in, 1 out]
                                n129 = Unbundle By Name(w337) -> ("status"=w332:bool)
                                n130 = Not(x=w332) -> (.not. x?=w333:bool)
                                n131 = case shown="False" w333 {
                                tunnel: w338 -> [_ w341]
                                tunnel: [w339 w340] -> w335
                                tunnel: w336 -> [w339 _]
                                frame False {
                                }
                                frame True {
                                n132 = call <vilib>:"Draw Flattened Pixmap.vi"("picture"=w341) -> ("new picture"=w340:picture)  [unwired: 8 in]
                                }
                                }
                                }
                                }
                                n133 = local write "Reagent pic 5"(w326) -> ()
                              }
                              frame #1 {
                                n134 = Wait (ms)(milliseconds to wait=100) -> ()  [unwired: 1 out]
                              }
                            }
                          }
                          frame #5 {
                            n135 = flat-sequence {
                              tunnel: w344 -> [w348]
                              tunnel: w343 -> [w347]
                              frame #0 {
                                n136 = local read "reagent name 4"() -> (w345:string)
                                n137 = String Length(string=w345) -> (length=w350:i32)
                                n138 = Greater Than 0?(x=w350) -> (x > 0?=w349:bool)
                                n139 = case shown="True" w349 {
                                tunnel: w347 -> [_ w356]
                                tunnel: w348 -> [w351 _]
                                tunnel: [w351 w355] -> w346
                                tunnel: w345 -> [_ w354]
                                frame False {
                                }
                                frame True {
                                n140 = call "Image_from_name.vi"("Chemical Name"=w354) -> ("error out"=w357:errorcluster, "Downloaded Picture"=w358:picture)  [unwired: 8 in, 1 out]
                                n141 = Unbundle By Name(w357) -> ("status"=w352:bool)
                                n142 = Not(x=w352) -> (.not. x?=w353:bool)
                                n143 = case shown="False" w353 {
                                tunnel: w358 -> [_ w361]
                                tunnel: [w359 w360] -> w355
                                tunnel: w356 -> [w359 _]
                                frame False {
                                }
                                frame True {
                                n144 = call <vilib>:"Draw Flattened Pixmap.vi"("picture"=w361) -> ("new picture"=w360:picture)  [unwired: 8 in]
                                }
                                }
                                }
                                }
                                n145 = local write "Reagent Pic 4"(w346) -> ()
                              }
                              frame #1 {
                                n146 = Wait (ms)(milliseconds to wait=100) -> ()  [unwired: 1 out]
                              }
                            }
                          }
                          frame #6 {
                            n147 = flat-sequence {
                              tunnel: w364 -> [w368]
                              tunnel: w363 -> [w367]
                              frame #0 {
                                n148 = local read "reagent  name 3"() -> (w365:string)
                                n149 = String Length(string=w365) -> (length=w370:i32)
                                n150 = Greater Than 0?(x=w370) -> (x > 0?=w369:bool)
                                n151 = case shown="True" w369 {
                                tunnel: w367 -> [_ w376]
                                tunnel: w368 -> [w371 _]
                                tunnel: [w371 w375] -> w366
                                tunnel: w365 -> [_ w374]
                                frame False {
                                }
                                frame True {
                                n152 = call "Image_from_name.vi"("Chemical Name"=w374) -> ("error out"=w377:errorcluster, "Downloaded Picture"=w378:picture)  [unwired: 8 in, 1 out]
                                n153 = Unbundle By Name(w377) -> ("status"=w372:bool)
                                n154 = Not(x=w372) -> (.not. x?=w373:bool)
                                n155 = case shown="False" w373 {
                                tunnel: w378 -> [_ w381]
                                tunnel: [w379 w380] -> w375
                                tunnel: w376 -> [w379 _]
                                frame False {
                                }
                                frame True {
                                n156 = call <vilib>:"Draw Flattened Pixmap.vi"("picture"=w381) -> ("new picture"=w380:picture)  [unwired: 8 in]
                                }
                                }
                                }
                                }
                                n157 = local write "Reagent Pic 3"(w366) -> ()
                              }
                              frame #1 {
                                n158 = Wait (ms)(milliseconds to wait=100) -> ()  [unwired: 1 out]
                              }
                            }
                          }
                        }
                      }
                      frame #3 {
                        n159 = local read "BAY 1"() -> (w393:u16)
                        n160 = local read "BAY 2"() -> (w392:u16)
                        n161 = local read "BAY 3"() -> (w391:u16)
                        n162 = local read "BAY 4"() -> (w390:u16)
                        n163 = local read "BAY 5"() -> (w389:u16)
                        n164 = local read "tube_id(in)"() -> (w400:enum16{".01", ".02", ".03", ".04"}[])
                        n165 = local read "Vr4"() -> (w403:dbl)
                        n166 = local read "tube_length(in)"() -> (w401:dbl[])
                        n167 = Build Array(w393, w392, w391, w390, w389) -> (w388:u16[])
                        n168 = local read "Vr3"() -> (w404:dbl)
                        n169 = local read "new_reactor_length"() -> (w398:bool[])
                        n170 = local read "Vr1"() -> (w406:dbl)
                        n171 = local read "Vr5"() -> (w402:dbl)
                        n172 = local read "Vr2"() -> (w405:dbl)
                        n173 = local read "new_reactor_volume"() -> (w396:bool[])
                        n174 = for {
                          N: 5 -> [_]
                          tunnel: w396 -> [w410] mode=indexing
                          tunnel: [w407] -> w394 mode=indexing
                          n175 = Select(t=1.0, s=w410, f=0.0) -> (s? t:f=w407:dbl)
                        }
                        n176 = for {
                          N: 5 -> [_]
                          tunnel: w398 -> [w414] mode=indexing
                          tunnel: [w411] -> w397 mode=indexing
                          n177 = Select(t=1.0, s=w414, f=0.0) -> (s? t:f=w411:dbl)
                        }
                        n178 = script code="tube_diameters = [.01,.02,.03,.04];\naddpath('C:\\Users\\HPLC\\Dropbox (MIT)\\MoD Files\\MATLAB');\ncalculate_reactor_volumes;"("BayConfig"=w388, "Vr1"=w406, "Vr2"=w405, "Vr3"=w404, "Vr4"=w403, "Vr5"=w402, "tube_length"=w401, "tube_id"=w400, "new_len_react"=w397, "new_vol_react"=w394) -> ("Vr1"=w387:dbl, "Vr2"=w386:dbl, "Vr3"=w385:dbl, "Vr4"=w384:dbl, "Vr5"=w383:dbl)  [unwired: 1 in, 1 out]
                        n179 = local write "Vr1"(w387) -> ()
                        n180 = local write "Vr2"(w386) -> ()
                        n181 = local write "Vr3"(w385) -> ()
                        n182 = local write "Vr4"(w384) -> ()
                        n183 = local write "Vr5"(w383) -> ()
                      }
                      frame #4 {
                        n184 = local read "Setup Error"() -> (w417:bool)
                        n185 = case shown="True" w417 {
                          tunnel: [TRUE FALSE] -> w415
                          tunnel: ["" "Sytem setup has not been confirmed!"] -> w416
                          frame False {
                          }
                          frame True {
                            n186 = local read "Error Message"() -> (w422:string)
                            n187 = One Button Dialog(message=w422) -> ()  [unwired: 1 in, 1 out]
                          }
                        }
                        n188 = local write "System Confirm Not Clicked"(w416) -> ()
                        n189 = local write "Setup Confirm"(w415) -> ()
                      }
                    }
                  }
                }
              }
            }
            n190 = local read "Stop"() -> (w201:bool)
            n191 = Or(x=w202, y=w201) -> (x .or. y?=w200:bool)
            n192 = disable-structure shown="Disabled" {
              disable-tunnel: 400 -> [w208 _]
              frame Disabled {
                n193 = event shown="[1]" {
                  selector: _ -> [_ _]
                  dyn-events: _ -> [_ _]
                  timeout: w208 -> [_ _]
                  event Timeout {
                    n194 = event-data() -> ()  [unwired: 1 in, 3 out]
                  }
                  event #1 (no event record) {
                    n195 = event-data() -> ()  [unwired: 1 in, 6 out]
                    n196 = local read "Setup Confirm"() -> (w209:bool)
                    n197 = local read "Reaction Scheme Confirm"() -> (w210:bool)
                    n198 = Not(x=w209) -> (.not. x?=w212:bool)
                    n199 = And(x=w210, y=w212) -> (x .and. y?=w211:bool)
                    n200 = case shown="True" w211 {
                      frame False {
                      }
                      frame True {
                        w214 = u16 0 items=["                     Bypass", "                Hot Reactor", "                 Separator"] ("BAY 5")
                        w215 = u16 0 items=["                     Bypass", "                Hot Reactor", "                  Separator"] ("BAY 4")
                        w216 = u16 0 items=["                     Bypass", "                 Hot Reactor", "                  Separator"] ("BAY 3")
                        w217 = u16 0 items=["                     Bypass", "                Hot Reactor", "                  Separator"] ("BAY 2")
                        w218 = u16 0 items=["                 Bypass", "             Hot Reactor", "               Separator"] ("BAY 1")
                        n201 = local write "BAY 3"(w216) -> ()
                        n202 = local write "BAY 4"(w215) -> ()
                        n203 = local write "BAY 5"(w214) -> ()
                        n204 = local write "BAY 2"(w217) -> ()
                        n205 = local write "BAY 1"(w218) -> ()
                        n206 = local write "Synthesis Route Array"(string[][] [["3-Br-Pyridine _ Biphenyl", "K2CO3", "PhB(OH)2", "", "", ""]] ("Synthesis Route Array")) -> ()
                      }
                    }
                  }
                }
              }
              frame Enabled {
              }
            }
            n207 = disable-structure shown="Disabled" {
              disable-tunnel: 400 -> [w204 _]
              frame Disabled {
                n208 = event shown="[1]" {
                  selector: _ -> [_ _]
                  dyn-events: _ -> [_ _]
                  timeout: w204 -> [_ _]
                  event Timeout {
                    n209 = event-data() -> ()  [unwired: 1 in, 3 out]
                  }
                  event #1 (no event record) {
                    n210 = event-data() -> ()  [unwired: 1 in, 6 out]
                    n211 = call "File Dialog"("prompt"="Load previously saved xml file") -> ("selected path"=w206:path)  [unwired: 11 in, 3 out]
                    n212 = Path To String(path=w206) -> (string=w205:string)
                    n213 = script code="xmlDoc = xmlread(file_path);\nroot = xmlDoc.getDocumentElement();\nb = root.getChildNodes;\nrecipe = b.getElementsByTagName('Bay1').item(0);"("file_path"=w205) -> ()  [unwired: 1 in, 1 out]
                  }
                }
              }
              frame Enabled {
              }
            }
          }
        }
        frame #1 {
          n214 = local read "Stop"() -> (w424:bool)
          n215 = Not(x=w424) -> (.not. x?=w423:bool)
          n216 = case shown="True" w423 {
            tunnel: w425 -> [_ w428]
            frame False {
              "stop_button clicked" <- TRUE ("stop_button clicked")
            }
            frame True {
              # "Parameters Initilization"
              n217 = flat-sequence {
                tunnel: w428 -> [w430]
                tunnel: [w429] -> w427
                tunnel: w427 -> [w589]
                frame #0 {
                  # "Setup bays(RFID - verify)"
                  n218 = disable-structure shown="Disabled" {
                    frame Disabled {
                      n219 = local read "BAY 1"() -> ()  [unwired: 1 out]
                      n220 = local read "BAY 2"() -> ()  [unwired: 1 out]
                      n221 = local read "BAY 3"() -> ()  [unwired: 1 out]
                      n222 = local read "BAY 4"() -> ()  [unwired: 1 out]
                      n223 = local read "BAY 5"() -> ()  [unwired: 1 out]
                    }
                    frame Enabled {
                    }
                  }
                }
                frame #1 {
                  n224 = while {
                    tunnel: w430 -> [w433]
                    tunnel: [w432] -> w429
                    stop <- w436 stop-if-true
                    n225 = flat-sequence {
                      tunnel: [w450] -> w432
                      tunnel: w433 -> [w531]
                      tunnel: [w449] -> w431
                      frame #0 {
                        n226 = while {
                          stop <- w440 stop-if-true
                          n227 = event shown="[1] \"System Parameters Confirm Button\": Value Change" {
                            selector: _ -> [_ _]
                            dyn-events: _ -> [_ _]
                            timeout: u32 200 ("milliseconds to wait") -> [_ _]
                            tunnel: [FALSE TRUE] -> w438
                            event Timeout {
                              n228 = event-data() -> ()  [unwired: 1 in, 3 out]
                            }
                            event "System Parameters Confirm Button": Value Change {
                              n229 = event-data() -> ()  [unwired: 1 in, 5 out]
                              n230 = local write "System Parameters Confirm Button"(FALSE) -> ()
                            }
                          }
                          n231 = Wait (ms)(milliseconds to wait=u32 500) -> ()  [unwired: 1 out]
                          n232 = local read "Stop"() -> (w441:bool)
                          n233 = Or(x=w441, y=w438) -> (x .or. y?=w440:bool)
                        }
                      }
                      frame #1 {
                        w470 = 0 ("disabled index (col)")
                        w482 = 1 ("disabled index (col)")
                        # "Do while parameters have not been correctly entered"
                        n234 = local read "Bay Parameters"() -> (w469:T2)
                        n235 = local read "Synthesis Route Array"() -> (w483:string[][])
                        n236 = local read "Total Number of Experiments"() -> (w502:dbl)
                        n237 = Unbundle By Name(w469) -> ("Continue from previous optimization?"=w530:bool)
                        n238 = Unbundle By Name(w469) -> ("Excel File Name"=w532:string)
                        n239 = Unbundle By Name(w469) -> ("Matlab File"=w528:string)
                        n240 = Unbundle By Name(w469) -> ("Bay 1.Run at set flowrate"=w574:bool)
                        n241 = Unbundle By Name(w469) -> ("Bay 1.Pump 1 Flowrate"=w580:dbl)
                        n242 = Unbundle By Name(w469) -> ("Bay 1.Pump 2 Flowrate"=w579:dbl)
                        n243 = Unbundle By Name(w469) -> ("Bay 2.Run at set flowrate"=w572:bool)
                        n244 = Unbundle By Name(w469) -> ("Bay 2.Pump 3 Flowrate"=w578:dbl)
                        n245 = Unbundle By Name(w469) -> ("Bay 3.Pump 4 Flowrate"=w577:dbl)
                        n246 = Unbundle By Name(w469) -> ("Bay 3.Run at set flowrate"=w571:bool)
                        n247 = Unbundle By Name(w469) -> ("Bay 4.Run at set flowrate"=w568:bool)
                        n248 = Unbundle By Name(w469) -> ("Bay 4.Pump 5 Flowrate"=w576:dbl)
                        n249 = Unbundle By Name(w469) -> ("Bay 5.Pump 6 Flowrate"=w575:dbl)
                        n250 = Unbundle By Name(w469) -> ("Bay 5.Run at set flowrate"=w567:bool)
                        n251 = Index Array(array=w483, index (row)=3, index (col)=w482) -> (element=w476:string)
                        n252 = Index Array(array=w483, index (row)=2, index (col)=w482) -> (element=w474:string)
                        n253 = Index Array(array=w483, index (row)=1, index (col)=w482) -> (element=w472:string)
                        n254 = Index Array(array=w483, index (row)=0, index (col)=w482) -> (element=w485:string)
                        n255 = Index Array(array=w483, index (row)=4, index (col)=w482) -> (element=w478:string)
                        n256 = Index Array(array=w483, index (row)=5, index (col)=w482) -> (element=w480:string)
                        n257 = Build Array(w485, w472, w474, w476, w478, w480) -> (w486:string[])
                        n258 = Index Array(array=w483, index (row)=0 ("index"), index (col)=w470) -> (element=w508:string)
                        n259 = for {
                          tunnel: w486 -> [w582] mode=indexing
                          tunnel: [w581] -> w471 mode=indexing
                          n260 = script code="ctemp1 = str2num(c_temp);"("c_temp"=w582) -> ("ctemp1"=w581:dbl)  [unwired: 1 in, 1 out]
                        }
                        n261 = Boolean To (0,1)(Boolean=w572) -> (0, 1=w527:i16)
                        n262 = Boolean To (0,1)(Boolean=w568) -> (0, 1=w569:i16)
                        n263 = Boolean To (0,1)(Boolean=w571) -> (0, 1=w570:i16)
                        n264 = Boolean To (0,1)(Boolean=w530) -> (0, 1=w529:i16)
                        n265 = Boolean To (0,1)(Boolean=w574) -> (0, 1=w573:i16)
                        n266 = Boolean To (0,1)(Boolean=w567) -> (0, 1=w566:i16)
                        n267 = Index Array(array=w483, index (row)=1 ("index"), index (col)=w470) -> (element=w503:string)
                        n268 = Index Array(array=w483, index (row)=2 ("index"), index (col)=w470) -> (element=w504:string)
                        n269 = Unbundle By Name(w469) -> ("Bay 1.optimize_temp"=w565:bool)
                        n270 = Unbundle By Name(w469) -> ("Bay 1.optimize_tau"=w563:bool)
                        n271 = Unbundle By Name(w469) -> ("Bay 2.optimize_temp"=w561:bool)
                        n272 = Unbundle By Name(w469) -> ("Bay 2.optimize_tau"=w559:bool)
                        n273 = Unbundle By Name(w469) -> ("Bay 3.optimize_temp"=w557:bool)
                        n274 = Unbundle By Name(w469) -> ("Bay 3.optimize_tau"=w555:bool)
                        n275 = Unbundle By Name(w469) -> ("Bay 4.optimize_temp"=w553:bool)
                        n276 = Unbundle By Name(w469) -> ("Bay 4.optimize_tau"=w551:bool)
                        n277 = Index Array(array=w483, index (row)=3 ("index"), index (col)=w470) -> (element=w505:string)
                        n278 = Boolean To (0,1)(Boolean=w553) -> (0, 1=w552:i16)
                        n279 = Boolean To (0,1)(Boolean=w551) -> (0, 1=w550:i16)
                        n280 = Index Array(array=w483, index (row)=4 ("index"), index (col)=w470) -> (element=w506:string)
                        n281 = Boolean To (0,1)(Boolean=w555) -> (0, 1=w554:i16)
                        n282 = Boolean To (0,1)(Boolean=w561) -> (0, 1=w560:i16)
                        n283 = Boolean To (0,1)(Boolean=w565) -> (0, 1=w564:i16)
                        n284 = Boolean To (0,1)(Boolean=w559) -> (0, 1=w558:i16)
                        n285 = Boolean To (0,1)(Boolean=w563) -> (0, 1=w562:i16)
                        n286 = Boolean To (0,1)(Boolean=w557) -> (0, 1=w556:i16)
                        n287 = Unbundle By Name(w469) -> ("Bay 5.optimize_temp"=w549:bool)
                        n288 = Unbundle By Name(w469) -> ("Bay 5.optimize_tau"=w547:bool)
                        n289 = Index Array(array=w483, index (row)=5 ("index"), index (col)=w470) -> (element=w507:string)
                        n290 = Boolean To (0,1)(Boolean=w549) -> (0, 1=w548:i16)
                        n291 = Boolean To (0,1)(Boolean=w547) -> (0, 1=w546:i16)
                        n292 = Build Array(w564, w562, w560, w558, w556, w554, w552, w550, w548, w546) -> (w545:i16[])
                        n293 = Unbundle By Name(w469) -> ("Bay 1.Temperature Params"=w542:dbl[])
                        n294 = Unbundle By Name(w469) -> ("Bay 2.Temperature Params"=w541:dbl[])
                        n295 = Unbundle By Name(w469) -> ("Bay 2.Resisdence time params"=w536:dbl[])
                        n296 = Unbundle By Name(w469) -> ("Bay 3.Temperature Params"=w540:dbl[])
                        n297 = Unbundle By Name(w469) -> ("Bay 3.Resisdence time params"=w535:dbl[])
                        n298 = Unbundle By Name(w469) -> ("Bay 4.Temperature Params"=w539:dbl[])
                        n299 = Unbundle By Name(w469) -> ("Bay 4.Resisdence time params"=w534:dbl[])
                        n300 = Unbundle By Name(w469) -> ("Bay 5.Temperature Params"=w538:dbl[])
                        n301 = Unbundle By Name(w469) -> ("Bay 5.Resisdence time params"=w533:dbl[])
                        n302 = Unbundle By Name(w469) -> ("Bay 1.pump params 2"=w501:dbl[])
                        n303 = Unbundle By Name(w469) -> ("Bay 1.pump params 1"=w537:dbl[])
                        n304 = Unbundle By Name(w469) -> ("Bay 1.Run at set temperature"=w492:bool)
                        n305 = Unbundle By Name(w469) -> ("Bay 2.Run at set temperature"=w490:bool)
                        n306 = Unbundle By Name(w469) -> ("Bay 3.Run at set temperature"=w489:bool)
                        n307 = Unbundle By Name(w469) -> ("Bay 4.Run at set temperature"=w488:bool)
                        n308 = Unbundle By Name(w469) -> ("Bay 5.Run at set temperature"=w487:bool)
                        n309 = Unbundle By Name(w469) -> ("Bay 3.Temperature"=w498:dbl)
                        n310 = Unbundle By Name(w469) -> ("Bay 1.Temperature"=w500:dbl)
                        n311 = Unbundle By Name(w469) -> ("Bay 2.Temperature"=w499:dbl)
                        n312 = Unbundle By Name(w469) -> ("Bay 4.Temperature"=w497:dbl)
                        n313 = Unbundle By Name(w469) -> ("Bay 5.Temperature"=w496:dbl)
                        n314 = Unbundle By Name(w469) -> ("Bay 3.pump_num_ratio"=w521:dbl)
                        n315 = Unbundle By Name(w469) -> ("Bay 4.pump_num_ratio"=w518:dbl)
                        n316 = Unbundle By Name(w469) -> ("Bay 5.pump_num_ratio"=w515:dbl)
                        n317 = Unbundle By Name(w469) -> ("Bay 2.pump_num_ratio"=w524:dbl)
                        n318 = Unbundle By Name(w469) -> ("Bay 4.pump_at_ratio"=w520:bool)
                        n319 = Boolean To (0,1)(Boolean=w520) -> (0, 1=w519:i16)
                        n320 = Unbundle By Name(w469) -> ("Bay 3.pump_at_ratio"=w523:bool)
                        n321 = Boolean To (0,1)(Boolean=w523) -> (0, 1=w522:i16)
                        n322 = Unbundle By Name(w469) -> ("Bay 5.pump_at_ratio"=w517:bool)
                        n323 = Boolean To (0,1)(Boolean=w517) -> (0, 1=w516:i16)
                        n324 = Unbundle By Name(w469) -> ("Bay 2.pump_at_ratio"=w526:bool)
                        n325 = Boolean To (0,1)(Boolean=w526) -> (0, 1=w525:i16)
                        n326 = Build Array(w500, w499, w498, w497, w496) -> (w495:dbl[])
                        n327 = Build Array(w492, w490, w489, w488, w487) -> (w491:bool[])
                        n328 = local read "Syringe_pump?"() -> (w448:bool)
                        n329 = for {
                          N: 5 -> [_]
                          tunnel: w491 -> [w586] mode=indexing
                          tunnel: [w585] -> w493 mode=indexing
                          n330 = Select(t=1.0, s=w586, f=0.0) -> (s? t:f=w585:dbl)
                        }
                        n331 = Unbundle By Name(w469) -> ("Internal Standard?"=w460:bool)
                        n332 = Unbundle By Name(w469) -> ("increas_decrease_hplc_peak"=w461:bool)
                        n333 = Unbundle By Name(w469) -> ("Hplc Wait time(min)"=w453:dbl)
                        n334 = Unbundle By Name(w469) -> ("Total Number of Experiments 2"=w452:dbl)
                        n335 = Unbundle By Name(w469) -> ("hplc_start"=w457:dbl)
                        n336 = Unbundle By Name(w469) -> ("ISTD start"=w455:dbl)
                        n337 = Unbundle By Name(w469) -> ("hplc_end"=w456:dbl)
                        n338 = Unbundle By Name(w469) -> ("throughput_yield"=w462:bool)
                        n339 = Unbundle By Name(w469) -> ("ISTD end"=w454:dbl)
                        n340 = Select(t=1.0, s=w448, f=0.0) -> (s? t:f=w447:dbl)
                        n341 = Select(t=1.0, s=w461, f=0.0) -> (s? t:f=w459:dbl)
                        n342 = Select(t=1.0, s=w460, f=0.0) -> (s? t:f=w458:dbl)
                        n343 = Select(t=0.0, s=w462, f=1.0) -> (s? t:f=w451:dbl)
                        n344 = script code="system_error = 0;\nnumPeaks = 1;\nstart_phase_time = 1;\nis_redo_exp = 0;\nFvalues = [];\nHPLC_Area = [];\n\nT1_span = [1 1]; T2_span = [1 1]; T3_span = [1 1]; T4_span = [1 1]; T5_span = [1 1];\nT_span = [T1_span;T2_span;T3_span;T4_span;T5_span];\n p1_span =  [1 1]; p2_span =  [1 1]; p3_span =  [1 1]; p4_span =  [1 1]; p5_span =  [1 1];  p6_span =  [1 1];\nOpt_params = [0 0 0 0 0 0 0 0 0 0 0];\nT_params = [T1_params;T2_params;T3_params;T4_params;T5_params];\npump_params = [pump1_params;pump2_params;pump3_params;pump4_params;pump5_params;pump6_params];\nopt_ctr = 0;ncall = 100;record_data = true;\nT1_SP = 23; T2_SP = 23; T3_SP = 23; T4_SP = 23; T5_SP = 23;\nT_span = [T1_span;T2_span;T3_span;T4_span;T5_span];\np_span = [p1_span;p2_span;p3_span;p4_span;p5_span;p6_span];\nno_errors = 1;\nP1 = 0; P2 =0; P3 = 0; P4 = 0; P5 = 0; P6 = 0;\nP = [P1, P2, P3,P4, P5, P6];\nis_first_set_of_exp = true;\nerror_message = 'System has no errors to report';\naddpath(genpath('C:\\Users\\HPLC\\Dropbox (MIT)\\MoD Files\\MATLAB'))\n%addpath(genpath('C:\\Users\\Admin\\Dropbox (MIT)\\MoD Files\\MATLAB'))\nallMSData = [];allHPLCData = [];allHPLCFile = [];\nBay_ratio = [0,Bay2_ratio,Bay3_ratio,Bay4_ratio,Bay5_ratio];\nBay_pump_ratio = [1, Bay2_pump_ratio, Bay3_pump_ratio, Bay4_pump_ratio, Bay5_pump_ratio];\nP_setrate = [P1_setrate, P2_setrate, P3_setrate, P4_setrate, P5_setrate, P6_setrate];\nuse_flowrate = [use_flowrate1, use_flowrate2,use_flowrate3, use_flowrate4, use_flowrate5];\npump_chem_name= []\nCurrExp = 1;\n% ****************************************************************************************************\n%Setup optimization\n   setup_optimization_params;\n   initialize_opt = 0;\n   nstop0 = 0;\n%*****************************************************************************************************\n% Setup excel and xml file writing\npath(path, pa);\nnumMSSig = 1;\nsetup_excel_output;\n%***************************************************************************************************\nredo = false;\nncall = ncall_in;"("use_flowrate1"=w573, "P1_setrate"=w580, "P2_setrate"=w579, "P3_setrate"=w578, "P4_setrate"=w577, "P5_setrate"=w576, "P6_setrate"=w575, "use_flowrate2"=w527, "use_flowrate3"=w570, "use_flowrate4"=w569, "use_flowrate5"=w566, "Optimize_params"=w545, "T1_params"=w542, "T2_params"=w541, "T3_params"=w540, "T4_params"=w539, "T5_params"=w538, "pump1_params"=w537, "pump3_params"=w536, "pump4_params"=w535, "pump5_params"=w534, "pump6_params"=w533, "xl_file"=w532, "pa"=w531, "Continue"=w529, "matlabsavefile"=w528, "Bay2_ratio"=w525, "Bay2_pump_ratio"=w524, "Bay3_ratio"=w522, "Bay3_pump_ratio"=w521, "Bay4_ratio"=w519, "Bay4_pump_ratio"=w518, "Bay5_ratio"=w516, "Bay5_pump_ratio"=w515, "pump1_chem"=w508, "pump6_chem"=w507, "pump5_chem"=w506, "pump4_chem"=w505, "pump3_chem"=w504, "pump2_chem"=w503, "Pump_concen"=w471, "ncall_in"=w502, "pump2_params"=w501, "T_SP"=w495, "Run_at_T_SP"=w493, "dcr_hplc_peak"=w459, "use_internal_std"=w458, "hplc_peak_start"=w457, "hplc_peak_end"=w456, "ISTD_start"=w455, "ISTD_end"=w454, "hplc_wait_time"=w453, "tot_num_exp"=w452, "throughput_yield"=w451, "syringe_pump"=w447) -> ("no_errors"=w544:dbl, "error_message"=w543:string)  [unwired: 1 in, 1 out]
                        n345 = Not Equal To 0?(x=w544) -> (x != 0?=w449:bool)
                        n346 = Not(x=w449) -> (.not. x?=w450:bool)
                        n347 = case shown="False" w450 {
                          tunnel: w543 -> [_ w588]
                          frame False {
                            n348 = local write "Setup Confirm 2"(TRUE ("Setup Confirm 2")) -> ()
                          }
                          frame True {
                            n349 = One Button Dialog(message=w588) -> ()  [unwired: 1 in, 1 out]
                          }
                        }
                      }
                    }
                    n350 = local read "Stop"() -> (w435:bool)
                    n351 = Or(x=w431, y=w435) -> (x .or. y?=w436:bool)
                    n352 = Wait (ms)(milliseconds to wait=u32 500) -> ()  [unwired: 1 out]
                  }
                }
                frame #2 {
                  n353 = local write "System Error"(w589) -> ()
                }
              }
            }
          }
        }
        frame #2 {
          # "Run Initial diagnostics"
        }
        frame #3 {
          # "Run System"
          n354 = while {
            tunnel: w590 -> [w1294]
            stop <- w1298 stop-if-true
            n355 = local read "running?"() -> (w1293:bool)
            n356 = local read "Temperature Control 1"() -> (w1295:bool)
            n357 = And(x=w1293, y=w1295) -> (x .and. y?=w1296:bool)
            n358 = case shown="True" w1296 {
              tunnel: w1294 -> [_ w1300]
              frame False {
                n359 = local write "Temp SS? 1"(TRUE ("Temp SS? 1")) -> ()
              }
              frame True {
                # "Bay 1 Temperature Controller"
                n360 = local read "Temperature SP 1"() -> (w1301:dbl)
                n361 = local read "Temperature 1"() -> (w1305:dbl)
                n362 = local read "SSR Duration 1"() -> (w1320:dbl)
                n363 = call-poly <vilib>:"PID Online Autotuning.vi"("setpoint"=w1301, "manipulated variable"=w1320, "autotuning parameters"=T9 {"type of controller"=enum."PID", "relay cycles"=3, "relay amplitude"=1.0, "control specifications"=enum."Normal", "PV noise level"=0.1} ("Autotuning Parameters R1"), "process variable"=w1305, "PID gains in"=T8 {"Proportional gain Kc"=0.38538, "Integral time Ti (sec)"=0.524375, "Derivative time Ti (sec)"=0.12585} ("PID gains 2")) -> ("setpoint out"=w1326:dbl, "process variable out"=w1325:dbl, "PID gains out"=w1322:T17)  [unwired: 6 in, 2 out]
                n364 = call <vilib>:"PID Autotuning (Temperature).vi"("desired temperature"=w1326, "measured temperature"=w1325, "plant parameters in"=w1322, "output range"=cluster{"output high":dbl, "output low":dbl} {"output high"=3.0, "output low"=-1.0} ("Output range")) -> ("output"=w1318:dbl)  [unwired: 12 in, 3 out]
                n365 = local write "SSR Duration 1"(w1318) -> ()
                n366 = Subtract(x=w1301, y=w1305) -> (x-y=w1312:dbl)
                n367 = Absolute Value(x=w1312) -> (abs(x)=w1315:dbl)
                n368 = Multiply(x=1000.0, y=w1318) -> (x*y=w1316:dbl)
                n369 = Greater Than 0?(x=w1316) -> (x > 0?=w1310:bool)
                n370 = Less Or Equal?(x=w1315, y=1.2) -> (x <= y?=w1313:bool)
                n371 = Greater?(x=w1301, y=w1305) -> (0:w1311:bool)
                n372 = And(x=w1310, y=w1311) -> (x .and. y?=w1308:bool)
                n373 = local write "Temp SS? 1"(w1313) -> ()
                n374 = Subtract(x=w1305, y=10.0) -> (x-y=w1306:dbl)
                n375 = Less?(x=w1306, y=w1301) -> (x < y?=w1309:bool)
                n376 = And(x=w1309, y=w1308) -> (x .and. y?=w1307:bool)
                n377 = case shown="True" w1307 {
                  tunnel: [errorcluster {"status"=FALSE, "code"=0, "source"=""} ("error out") w1336] -> _
                  tunnel: 2 -> [_ w1333]
                  tunnel: w1316 -> [w1330 w1334]
                  tunnel: [0.0 w1338] -> w1303
                  tunnel: w1301 -> [_ w1337]
                  tunnel: w1300 -> [_ w1335]
                  frame False {
                    n378 = Absolute Value(x=w1330) -> (abs(x)=w1331:dbl)
                    n379 = Wait (ms)(milliseconds to wait=w1331) -> ()  [unwired: 1 out]
                  }
                  frame True {
                    n380 = call "TurnOnRelayArduino.vi"("channel"=w1333, "duration"=w1334, "LINX Resource"=w1335) -> ("error out"=w1336:errorcluster)  [unwired: 7 in, 1 out]
                    n381 = script code="tempdiff1= SP1 - T1;\nif tempdiff1 > 10\n  if slope1 < .01\n     temp_check1 = temp_check1 + 1;\n  else\n      temp_check1 =0;\n  end\nend\n\nif temp_check1 > 9\n  temp_error1 = 1\nend"("SP1"=w1337) -> ("temp_error1"=w1338:dbl)  [unwired: 1 in, 1 out]
                  }
                }
                n382 = Not Equal To 0?(x=w1303) -> (x != 0?=w1302:bool)
                n383 = case shown="True" w1302 {
                  frame False {
                  }
                  frame True {
                    n384 = local write "Error Message"("Bay 1 Temperature Heating Error") -> ()
                  }
                }
                n385 = case shown="True" w1302 {
                  tunnel: w1302 -> [_ w1328]
                  frame False {
                  }
                  frame True {
                    n386 = local write "System Error"(w1328) -> ()
                    n387 = local write "Stop"(w1328) -> ()
                  }
                }
              }
            }
            n388 = Wait (ms)(milliseconds to wait=u32 400) -> ()  [unwired: 1 out]
            n389 = local read "Stop"() -> (w1298:bool)
          }
          n390 = local read "Bay Parameters"() -> (w594:T2)
          n391 = while {
            tunnel: w590 -> [w1248]
            stop <- w1252 stop-if-true
            n392 = local read "running?"() -> (w1247:bool)
            n393 = local read "Temperature Control 2"() -> (w1249:bool)
            n394 = And(x=w1247, y=w1249) -> (x .and. y?=w1250:bool)
            n395 = case shown="True" w1250 {
              tunnel: w1248 -> [_ w1254]
              frame False {
                n396 = local write "Temp SS? 2"(TRUE ("Temp SS? 2")) -> ()
              }
              frame True {
                # "Bay 2 Temperature Controller"
                n397 = local read "Temperature SP 2"() -> (w1256:dbl)
                n398 = local read "Temperature 2"() -> (w1259:dbl)
                n399 = local read "SSR Duration 2"() -> (w1277:dbl)
                n400 = call-poly <vilib>:"PID Online Autotuning.vi"("setpoint"=w1256, "manipulated variable"=w1277, "autotuning parameters"=T9 {"type of controller"=enum."PID", "relay cycles"=3, "relay amplitude"=1.0, "control specifications"=enum."Normal", "PV noise level"=0.1} ("Autotuning Parameters R1"), "process variable"=w1259, "PID gains in"=T8 {"Proportional gain Kc"=0.38538, "Integral time Ti (sec)"=0.524375, "Derivative time Ti (sec)"=0.12585} ("PID gains 2")) -> ("setpoint out"=w1275:dbl, "process variable out"=w1274:dbl, "PID gains out"=w1280:T17)  [unwired: 6 in, 2 out]
                n401 = call <vilib>:"PID Autotuning (Temperature).vi"("desired temperature"=w1275, "measured temperature"=w1274, "plant parameters in"=w1280, "output range"=cluster{"output high":dbl, "output low":dbl} {"output high"=3.0, "output low"=-1.0} ("Output range")) -> ("output"=w1270:dbl)  [unwired: 12 in, 3 out]
                n402 = local write "SSR Duration 2"(w1270) -> ()
                n403 = Greater?(x=w1256, y=w1259) -> (0:w1265:bool)
                n404 = Multiply(x=1000.0, y=w1270) -> (x*y=w1272:dbl)
                n405 = Greater Than 0?(x=w1272) -> (x > 0?=w1264:bool)
                n406 = And(x=w1264, y=w1265) -> (x .and. y?=w1262:bool)
                n407 = Subtract(x=w1256, y=w1259) -> (x-y=w1267:dbl)
                n408 = Absolute Value(x=w1267) -> (abs(x)=w1269:dbl)
                n409 = Subtract(x=w1259, y=10.0) -> (x-y=w1261:dbl)
                n410 = Less Or Equal?(x=w1269, y=1.2) -> (x <= y?=w1266:bool)
                n411 = local write "Temp SS? 2"(w1266) -> ()
                n412 = Less?(x=w1261, y=w1256) -> (x < y?=w1263:bool)
                n413 = And(x=w1263, y=w1262) -> (x .and. y?=w1258:bool)
                n414 = case shown="True" w1258 {
                  tunnel: [errorcluster {"status"=FALSE, "code"=0, "source"=""} ("error out") w1290] -> _
                  tunnel: 3 -> [_ w1287]
                  tunnel: w1272 -> [w1284 w1288]
                  tunnel: [0.0 w1292] -> w1257
                  tunnel: w1256 -> [_ w1291]
                  tunnel: w1254 -> [_ w1289]
                  frame False {
                    n415 = Absolute Value(x=w1284) -> (abs(x)=w1285:dbl)
                    n416 = Wait (ms)(milliseconds to wait=w1285) -> ()  [unwired: 1 out]
                  }
                  frame True {
                    n417 = call "TurnOnRelayArduino.vi"("channel"=w1287, "duration"=w1288, "LINX Resource"=w1289) -> ("error out"=w1290:errorcluster)  [unwired: 7 in, 1 out]
                    n418 = script code="tempdiff2= SP2 - T2;\nif tempdiff2 > 10\n  if slope2 < .01\n     temp_check2 = temp_check2 + 1;\n  else\n      temp_check2 =0;\n  end\nend\n\nif temp_check2 > 9\n  temp_error2 = 1\nend"("SP2"=w1291) -> ("temp_error2"=w1292:dbl)  [unwired: 1 in, 1 out]
                  }
                }
                n419 = Not Equal To 0?(x=w1257) -> (x != 0?=w1255:bool)
                n420 = case shown="True" w1255 {
                  frame False {
                  }
                  frame True {
                    n421 = local write "Error Message"("Bay 2 Temperature Heating Error") -> ()
                  }
                }
                n422 = case shown="True" w1255 {
                  tunnel: w1255 -> [_ w1282]
                  frame False {
                  }
                  frame True {
                    n423 = local write "Stop"(w1282) -> ()
                    n424 = local write "System Error"(w1282) -> ()
                  }
                }
              }
            }
            n425 = local read "Stop"() -> (w1252:bool)
            n426 = Wait (ms)(milliseconds to wait=u32 400) -> ()  [unwired: 1 out]
          }
          n427 = local read "Stop"() -> (w591:bool)
          n428 = Not(x=w591) -> (.not. x?=w593:bool)
          n429 = case shown="True" w593 {
            tunnel: w594 -> [_ w599]
            tunnel: w592 -> [_ w598]
            tunnel: w590 -> [_ w597]
            frame False {
            }
            frame True {
              n430 = while {
                tunnel: w599 -> [w613]
                tunnel: w598 -> [w605]
                tunnel: w597 -> [w600]
                i -> [w612]
                stop <- w606 stop-if-true
                n431 = local read "running?"() -> (w601:bool)
                n432 = Wait (ms)(milliseconds to wait=u32 1000) -> ()  [unwired: 1 out]
                n433 = Increment(x=w612) -> (x+1=w602:i32)
                n434 = case shown="True" w601 {
                  tunnel: w612 -> [w618 _]
                  tunnel: w613 -> [_ _]
                  tunnel: [w620 w624] -> w603
                  tunnel: [0.0 w625] -> w608
                  tunnel: w605 -> [_ w623]
                  tunnel: w600 -> [_ w621]
                  frame False {
                    # "STANDBY MODE"
                    n435 = Add(x=w618, y=2.0) -> (x+y=w620:dbl)
                  }
                  frame True {
                    n436 = flat-sequence {
                      tunnel: w623 -> [w627]
                      tunnel: [w627] -> w622
                      tunnel: [w637] -> w625
                      tunnel: [200.0] -> w624
                      tunnel: w622 -> [w635]
                      tunnel: w621 -> [w629]
                      frame #0 {
                        n437 = local write "stop_xl_write"(FALSE ("stop_xl_write")) -> ()
                      }
                      frame #1 {
                        # "Increase flowrate of dilution stream"
                        # "Wait mixed stream reaches SL"
                        # "SNOBFIT"
                        # "Optimize"
                        # "Run Experimental Conditions"
                        # "Optimize/Synthesize"
                        n438 = local read "Syringe_pump?"() -> (w628:bool)
                        n439 = local read "Stop"() -> (w632:bool)
                        n440 = Not(x=w632) -> (.not. x?=w631:bool)
                        n441 = case shown="True" w631 {
                          tunnel: [1.0 w660] -> w640
                          tunnel: [w648 w659] -> w634
                          tunnel: [0.0 w658] -> w633
                          tunnel: [w648 w657] -> w630
                          tunnel: w628 -> [_ w654]
                          frame False {
                            w648 = dbl[] []
                          }
                          frame True {
                            n442 = Select(t=1.0, s=w654, f=0.0) -> (s? t:f=w653:dbl)
                            n443 = script code="optimization_main_loop"("syringe_pump"=w653) -> ("Conditions_Array"=w659:dbl[], "opt_ctr"=w660:dbl, "P_tot"=w658:dbl, "tau_array"=w657:dbl[], "experiment_history"=w655:dbl[][])  [unwired: 1 in, 1 out]
                            n444 = call-poly <vilib>:"Array To Matrix.vi"("Real 2D Array"=w655) -> ("Real Matrix"=w656:T18)
                            n445 = local write "experiment history"(w656) -> ()
                          }
                        }
                        "P_tot" <- w633
                        n446 = local read "COMM Port :: Milligat Pumps"() -> (w641:refnum<visa-resource-name>)
                        n447 = Equal?(x=w640, y=1.0) -> (x = y?=w638:bool)
                        n448 = flat-sequence {
                          tunnel: w634 -> [w1092]
                          tunnel: w630 -> [w1086]
                          frame #0 {
                            # "Start recording data"
                            n449 = Index Array(array=w1092, index=5) -> (element=w1104:dbl)
                            n450 = Index Array(array=w1092, index=0) -> (element=w1099:dbl)
                            n451 = Index Array(array=w1092, index=1) -> (element=w1100:dbl)
                            n452 = Index Array(array=w1092, index=2) -> (element=w1102:dbl)
                            n453 = Index Array(array=w1092, index=3) -> (element=w1101:dbl)
                            n454 = Index Array(array=w1092, index=4) -> (element=w1103:dbl)
                            n455 = local write "Pump setpoint(ul/min) 2"(w1100) -> ()
                            n456 = local write "Pump setpoint(ul/min) 4"(w1102) -> ()
                            n457 = local write "Pump setpoint(ul/min) 5"(w1103) -> ()
                            n458 = local write "Pump setpoint(ul/min) 3"(w1101) -> ()
                            n459 = local write "Pump setpoint(ul/min) 6"(w1104) -> ()
                            n460 = local write "Pump setpoint(ul/min) 1"(w1099) -> ()
                            n461 = Index Array(array=w1086, index=0) -> (element=w1091:dbl)
                            n462 = Index Array(array=w1086, index=4) -> (element=w1090:dbl)
                            n463 = Index Array(array=w1086, index=3) -> (element=w1089:dbl)
                            n464 = Index Array(array=w1086, index=2) -> (element=w1088:dbl)
                            n465 = Index Array(array=w1086, index=1) -> (element=w1087:dbl)
                            n466 = local write "tau 2"(w1087) -> ()
                            n467 = local write "tau 3"(w1088) -> ()
                            n468 = local write "tau 4"(w1089) -> ()
                            n469 = local write "tau 5"(w1090) -> ()
                            n470 = local write "tau 1"(w1091) -> ()
                          }
                        }
                        n471 = flat-sequence {
                          tunnel: w641 -> [w664]
                          tunnel: w634 -> [w663]
                          tunnel: w638 -> [w662]
                          tunnel: [w662] -> w647
                          tunnel: w635 -> [w661]
                          tunnel: w647 -> [w808]
                          tunnel: [w808] -> w646
                          tunnel: w646 -> [w828]
                          tunnel: [w826] -> w645
                          tunnel: w634 -> [w852]
                          tunnel: w645 -> [w851]
                          tunnel: w629 -> [w850]
                          tunnel: [w1022] -> w644
                          tunnel: w644 -> [w1035]
                          tunnel: [w1035] -> w643
                          tunnel: w643 -> [w1043]
                          tunnel: [w1043] -> w642
                          tunnel: [w1080] -> w637
                          tunnel: w642 -> [w1080]
                          frame #0 {
                            # "Setup pump flowrates and temperature setpoints"
                            n472 = stacked-sequence {
                              tunnel: w664 -> [w686 _ _ _ _]
                              tunnel: w664 -> [_ w726 _ _ _]
                              tunnel: w664 -> [_ _ w750 _ _]
                              tunnel: w664 -> [_ _ _ w774 _]
                              tunnel: w664 -> [_ _ _ _ w798]
                              tunnel: w663 -> [w683 w724 w748 w772 w795]
                              tunnel: w662 -> [w673 w717 w741 w765 w789]
                              tunnel: w661 -> [w671 _ _ _ _]
                              frame #0 {
                                # "Bay 1"
                                n473 = local read "Syringe_pump?"() -> (w672:bool)
                                n474 = Index Array(array=w683, index=0) -> (element=w681:dbl)
                                n475 = local read "BAY 1"() -> (w666:u16)
                                n476 = Index Array(array=w683, index=1) -> (element=w680:dbl)
                                n477 = Index Array(array=w683, index=6) -> (element=w679:dbl)
                                n478 = script code="MATLAB script"("T1_SP"=w679) -> ()  [unwired: 1 in, 1 out]
                                n479 = Less Or Equal?(x=w666, y=u16 4) -> (x <= y?=w668:bool)
                                n480 = Greater Or Equal?(x=w666, y=u16 1) -> (x >= y?=w669:bool)
                                n481 = And(x=w669, y=w668) -> (x .and. y?=w670:bool)
                                n482 = Greater Than 0?(x=w681) -> (x > 0?=w678:bool)
                                n483 = And(x=w678, y=w673) -> (x .and. y?=w677:bool)
                                n484 = Greater Than 0?(x=w680) -> (x > 0?=w676:bool)
                                n485 = And(x=w676, y=w673) -> (x .and. y?=w675:bool)
                                n486 = And(x=w670, y=w673) -> (x .and. y?=w674:bool)
                                n487 = case shown="False" w672 {
                                tunnel: w686 -> [w689 _]
                                tunnel: w680 -> [w688 w694]
                                tunnel: w675 -> [w687 w695]
                                tunnel: w671 -> [_ w693]
                                frame False {
                                n488 = case shown="False" w687 {
                                tunnel: w689 -> [w691 _]
                                tunnel: w688 -> [w690 _]
                                frame False {
                                n489 = call "PumpDispense.vi"("Flowrate(ul/min)"=w690, "Pump Address"="j", "Pump COMM Port"=w691) -> ()  [unwired: 7 in, 2 out]
                                }
                                frame True {
                                }
                                }
                                }
                                frame True {
                                n490 = case shown="False" w695 {
                                tunnel: w694 -> [_ w697]
                                tunnel: w693 -> [w696 w698]
                                frame False {
                                n491 = call <instrlib>:"Stop Pump.vi"("VISA resource name"=w696) -> ()  [unwired: 9 in, 2 out]
                                }
                                frame True {
                                w699 = u16 0 items=["Infuse", "Withdraw"] ("Run Direction (0:Infuse)")
                                w700 = u32 4 items=["milliliters per hour (ml/hr)", "milliliters per minute (ml/min)", "milliliters per second (ml/sec)", "microliters per hour (ul/hr)", "microliters per minute (ul/min)", "microliters per second (ul/sec)", "nanoliters per hour (nl/hr)", "nanoliters per minute (nl/min)", "nanoliters per second (nl/sec)", "picoliters per hour (pl/hr)", "picoliters per minute (pl/min)", "picoliters per second (pl/sec)"] ("Flow Rate Units (1:ml/min)")
                                w701 = u16 0 items=["Infuse", "Withdraw"] ("Pump Direction (0:Infuse)")
                                n492 = call <instrlib>:"Configure Flow Rate & Direction.vi"("VISA resource name"=w698, "Pump Direction (0:Infuse)"=w701, "Flow Rate (5.00)"=w697, "Flow Rate Units (1:ml/min)"=w700) -> ("VISA resource name out"=w702:refnum<visa-resource-name>)  [unwired: 10 in, 1 out]
                                n493 = call <instrlib>:"Start Pump.vi"("Run Direction (0:Infuse)"=w699, "VISA resource name"=w702) -> ()  [unwired: 8 in, 2 out]
                                }
                                }
                                }
                                }
                                n494 = case shown="False" w677 {
                                tunnel: w686 -> [w706 w708]
                                tunnel: w681 -> [_ w709]
                                frame False {
                                n495 = call "PumpStop.vi"("Pump Address"="g", "Pump COMM Port"=w706) -> ()  [unwired: 9 in, 1 out]
                                }
                                frame True {
                                n496 = call "PumpDispense.vi"("Flowrate(ul/min)"=w709, "Pump Address"="g", "Pump COMM Port"=w708) -> ()  [unwired: 7 in, 2 out]
                                }
                                }
                                n497 = case shown="True" w674 {
                                tunnel: w679 -> [_ w705]
                                frame False {
                                n498 = local write "Temperature Control 1"(FALSE) -> ()
                                }
                                frame True {
                                n499 = local write "Temperature SP 1"(w705) -> ()
                                n500 = local write "Temperature Control 1"(TRUE ("Temperature Control 1")) -> ()
                                }
                                }
                              }
                              frame #1 {
                                # "Bay 2"
                                n501 = local read "BAY 2"() -> (w713:u16)
                                n502 = Index Array(array=w724, index=2) -> (element=w721:dbl)
                                n503 = Index Array(array=w724, index=7) -> (element=w722:dbl)
                                n504 = script code="MATLAB script"("T2_SP"=w722) -> ()  [unwired: 1 in, 1 out]
                                n505 = Greater Than 0?(x=w721) -> (x > 0?=w719:bool)
                                n506 = And(x=w719, y=w717) -> (x .and. y?=w718:bool)
                                n507 = Greater Or Equal?(x=w713, y=u16 1) -> (x >= y?=w711:bool)
                                n508 = Less Or Equal?(x=w713, y=u16 4) -> (x <= y?=w716:bool)
                                n509 = And(x=w711, y=w716) -> (x .and. y?=w715:bool)
                                n510 = And(x=w715, y=w717) -> (x .and. y?=w720:bool)
                                n511 = case shown="True" w720 {
                                tunnel: w722 -> [_ w733]
                                frame False {
                                n512 = local write "Temperature Control 2"(FALSE) -> ()
                                }
                                frame True {
                                n513 = local write "Temperature Control 2"(TRUE ("Temperature Control 2")) -> ()
                                n514 = local write "Temperature SP 2"(w733) -> ()
                                }
                                }
                                n515 = case shown="False" w718 {
                                tunnel: w721 -> [_ w729]
                                tunnel: w726 -> [w727 w730]
                                frame False {
                                n516 = call "PumpStop.vi"("Pump Address"="i", "Pump COMM Port"=w727) -> ()  [unwired: 9 in, 1 out]
                                }
                                frame True {
                                n517 = call "PumpDispense.vi"("Flowrate(ul/min)"=w729, "Pump Address"="i", "Pump COMM Port"=w730) -> ()  [unwired: 7 in, 2 out]
                                }
                                }
                              }
                              frame #2 {
                                # "Bay 3"
                                n518 = local read "BAY 3"() -> (w736:u16)
                                n519 = Index Array(array=w748, index=3) -> (element=w745:dbl)
                                n520 = Not Equal To 0?(x=w745) -> (x != 0?=w744:bool)
                                n521 = Index Array(array=w748, index=8) -> (element=w746:dbl)
                                n522 = script code="MATLAB script"("T3_SP"=w746) -> ()  [unwired: 1 in, 1 out]
                                n523 = Less Or Equal?(x=w736, y=u16 4) -> (x <= y?=w740:bool)
                                n524 = Greater Or Equal?(x=w736, y=u16 1) -> (x >= y?=w737:bool)
                                n525 = And(x=w737, y=w740) -> (x .and. y?=w735:bool)
                                n526 = And(x=w735, y=w741) -> (x .and. y?=w742:bool)
                                n527 = And(x=w744, y=w741) -> (x .and. y?=w743:bool)
                                n528 = case shown="True" w743 {
                                tunnel: w745 -> [_ w753]
                                tunnel: w750 -> [w751 w754]
                                frame False {
                                n529 = call "PumpStop.vi"("Pump Address"="e", "Pump COMM Port"=w751) -> ()  [unwired: 9 in, 1 out]
                                }
                                frame True {
                                n530 = call "PumpDispense.vi"("Flowrate(ul/min)"=w753, "Pump Address"="e", "Pump COMM Port"=w754) -> ()  [unwired: 7 in, 2 out]
                                }
                                }
                                n531 = case shown="False" w742 {
                                tunnel: w746 -> [_ w757]
                                frame False {
                                n532 = local write "Temperature Control 3"(FALSE) -> ()
                                }
                                frame True {
                                n533 = local write "Temperature Control 3"(TRUE ("Temperature Control 3")) -> ()
                                n534 = local write "Temperature SP 3"(w757) -> ()
                                }
                                }
                              }
                              frame #3 {
                                # "Bay 4"
                                n535 = Index Array(array=w772, index=9) -> (element=w769:dbl)
                                n536 = script code="MATLAB script"("T4_SP"=w769) -> ()  [unwired: 1 in, 1 out]
                                n537 = Index Array(array=w772, index=4) -> (element=w770:dbl)
                                n538 = Not Equal To 0?(x=w770) -> (x != 0?=w768:bool)
                                n539 = local read "BAY 4"() -> (w759:u16)
                                n540 = And(x=w768, y=w765) -> (x .and. y?=w767:bool)
                                n541 = Less Or Equal?(x=w759, y=u16 4) -> (x <= y?=w764:bool)
                                n542 = Greater Or Equal?(x=w759, y=u16 1) -> (x >= y?=w761:bool)
                                n543 = And(x=w761, y=w764) -> (x .and. y?=w760:bool)
                                n544 = And(x=w760, y=w765) -> (x .and. y?=w766:bool)
                                n545 = case shown="True" w767 {
                                tunnel: w774 -> [w775 w778]
                                tunnel: w770 -> [_ w777]
                                frame False {
                                n546 = call "PumpStop.vi"("Pump Address"="f", "Pump COMM Port"=w775) -> ()  [unwired: 9 in, 1 out]
                                }
                                frame True {
                                n547 = call "PumpDispense.vi"("Flowrate(ul/min)"=w777, "Pump Address"="f", "Pump COMM Port"=w778) -> ()  [unwired: 7 in, 2 out]
                                }
                                }
                                n548 = case shown="True" w766 {
                                tunnel: w769 -> [_ w781]
                                frame False {
                                n549 = local write "Temperature Control 4"(FALSE ("Temperature Control 4")) -> ()
                                }
                                frame True {
                                n550 = local write "Temperature SP 4"(w781) -> ()
                                n551 = local write "Temperature Control 4"(TRUE ("Temperature Control 5")) -> ()
                                }
                                }
                              }
                              frame #4 {
                                # "Bay 5"
                                n552 = Index Array(array=w795, index=5) -> (element=w793:dbl)
                                n553 = Index Array(array=w795, index=4) -> (element=w794:dbl)
                                n554 = script code="MATLAB script"("T5_SP"=w794) -> ()  [unwired: 1 in, 1 out]
                                n555 = local read "BAY 5"() -> (w784:u16)
                                n556 = Not Equal To 0?(x=w793) -> (x != 0?=w791:bool)
                                n557 = And(x=w791, y=w789) -> (x .and. y?=w790:bool)
                                n558 = Less Or Equal?(x=w784, y=u16 4) -> (x <= y?=w788:bool)
                                n559 = Greater Or Equal?(x=w784, y=u16 1) -> (x >= y?=w785:bool)
                                n560 = case shown="False" w790 {
                                tunnel: w798 -> [w799 w802]
                                tunnel: w793 -> [_ w801]
                                frame False {
                                n561 = call "PumpStop.vi"("Pump Address"="h", "Pump COMM Port"=w799) -> ()  [unwired: 9 in, 1 out]
                                }
                                frame True {
                                n562 = call "PumpDispense.vi"("Flowrate(ul/min)"=w801, "Pump Address"="h", "Pump COMM Port"=w802) -> ()  [unwired: 7 in, 2 out]
                                }
                                }
                                n563 = And(x=w785, y=w788) -> (x .and. y?=w783:bool)
                                n564 = And(x=w783, y=w789) -> (x .and. y?=w792:bool)
                                n565 = case shown="True" w792 {
                                tunnel: w794 -> [_ w805]
                                frame False {
                                n566 = local write "Temperature Control 5"(FALSE ("Temperature Control 5")) -> ()
                                }
                                frame True {
                                n567 = local write "Temperature SP 5"(w805) -> ()
                                n568 = local write "Temperature Control 5"(TRUE ("Temperature Control 5")) -> ()
                                }
                                }
                              }
                            }
                          }
                          frame #1 {
                            # "Wait till Steady State temperature readings on all bays"
                            n569 = while {
                              tunnel: w808 -> [w809]
                              stop <- w810 stop-if-true
                              n570 = flat-sequence {
                                tunnel: [w813] -> w810
                                tunnel: w809 -> [w812]
                                frame #0 {
                                n571 = Wait (ms)(milliseconds to wait=u32 1500) -> ()  [unwired: 1 out]
                                }
                                frame #1 {
                                n572 = local read "Temp SS? 2"() -> (w816:bool)
                                n573 = local read "Temp SS? 3"() -> (w817:bool)
                                n574 = local read "Temp SS? 4"() -> (w818:bool)
                                n575 = local read "Temp SS? 5"() -> (w819:bool)
                                n576 = local read "Temp SS? 1"() -> (w815:bool)
                                n577 = Not(x=w812) -> (.not. x?=w825:bool)
                                n578 = local read "Stop"() -> (w814:bool)
                                n579 = And(x=w817, y=w818) -> (x .and. y?=w821:bool)
                                n580 = And(x=w815, y=w816) -> (x .and. y?=w822:bool)
                                n581 = And(x=w822, y=w821) -> (x .and. y?=w820:bool)
                                n582 = And(x=w820, y=w819) -> (x .and. y?=w823:bool)
                                n583 = Or(x=w825, y=w823) -> (x .or. y?=w824:bool)
                                n584 = Or(x=w824, y=w814) -> (x .or. y?=w813:bool)
                                }
                              }
                            }
                            n585 = local write "Calculate condition"(TRUE ("Calculate condition")) -> ()
                          }
                          frame #2 {
                            n586 = flat-sequence {
                              tunnel: w828 -> [w830]
                              tunnel: [w830] -> w827
                              tunnel: w827 -> [w837]
                              tunnel: [w837] -> w826
                              frame #0 {
                                n587 = local write "Equlibrating Temperature"(TRUE) -> ()
                              }
                              frame #1 {
                                # "Wait 1.5 system volumes"
                                n588 = local read "Number of System Flushes per condtion"() -> (w834:dbl)
                                n589 = local read "Extra system dead volume"() -> (w835:dbl)
                                n590 = script code="start = tic;\nP_tot = P1+P2+P3+P4+P5+P6;\nif P_tot >0\n  extra_res = extr_sys_dead_vol/P_tot;\nelse\n   extra_res =0;\nend\ntotal_sys_res = tau1 + tau2 + tau3 + tau4 + tau5 + extra_res;\ntotal_wait_time = total_sys_res*num_flush_per_cond*60;"("extr_sys_dead_vol"=w835, "num_flush_per_cond"=w834) -> ("??"=w838:errorcluster, "total_wait_time"=w832:dbl, "total_sys_res"=→"Total System Resisdence Time(min)":dbl)  [unwired: 1 in]
                                n591 = Divide(x=w832, y=60.0) -> (x/y=→"total_flush_time":dbl)
                                n592 = while {
                                tunnel: w837 -> [w840]
                                tunnel: w838 -> [w843]
                                stop <- w844 stop-if-true
                                # "Check if system is flushed every 10 seconds"
                                n593 = script code="end1 = toc(start);\nflush_time = 0;\nif end1 > total_wait_time\n   flush_time = 1;\nend\ncurr_wait_time = end1 /60;"("??"=w843) -> ("flush_time"=w847:dbl, "curr_wait_time"=w842:dbl)  [unwired: 1 out]
                                "curr_wait_time" <- w842
                                n594 = Not Equal To 0?(x=w847) -> (x != 0?=w846:bool)
                                n595 = Multiply(x=60.0, y=w842) -> ()  [unwired: 1 out]
                                n596 = local read "Stop"() -> (w849:bool)
                                n597 = Or(x=w846, y=w849) -> (x .or. y?=w845:bool)
                                n598 = Not(x=w840) -> (.not. x?=w839:bool)
                                n599 = Wait (ms)(milliseconds to wait=u32 10000) -> ()  [unwired: 1 out]
                                n600 = Or(x=w845, y=w839) -> (x .or. y?=w844:bool)
                                }
                              }
                            }
                          }
                          frame #3 {
                            # "Collect HPLC Data"
                            n601 = flat-sequence {
                              tunnel: w852 -> [w861]
                              tunnel: w851 -> [w860]
                              tunnel: w850 -> [w859]
                              tunnel: w850 -> [w858]
                              frame #0 {
                                n602 = local read "pause for ms"() -> (w855:bool)
                                n603 = case shown="True" w855 {
                                frame False {
                                }
                                frame True {
                                n604 = One Button Dialog(message="Press OK to Analyze Data", button name ("OK")="OK" ("Left Button Text (\"Yes\")")) -> ()  [unwired: 1 out]
                                }
                                }
                                n605 = local write "Flushing System"(TRUE ("Flushing System")) -> ()
                                "System Flushed?" <- TRUE ("System Flushed?")
                              }
                              frame #1 {
                                n606 = flat-sequence {
                                tunnel: w861 -> [w866]
                                tunnel: w860 -> [_]
                                tunnel: w859 -> [w865]
                                tunnel: w858 -> [w864]
                                frame #0 {
                                }
                                frame #1 {
                                n607 = flat-sequence {
                                tunnel: w866 -> [w867]
                                tunnel: w865 -> [w939]
                                tunnel: w866 -> [_]
                                tunnel: [w959] -> w863
                                tunnel: [w958] -> w862
                                tunnel: w864 -> [w957]
                                tunnel: w863 -> [w992]
                                tunnel: w862 -> [w991]
                                frame #0 {
                                n608 = local read "COMM Port :: Milligat Pumps"() -> (w869:refnum<visa-resource-name>)
                                n609 = stacked-sequence {
                                tunnel: w869 -> [w872 w884 w902 w907 w916 w929]
                                tunnel: w867 -> [w871 w880 w899 w909 w918 w925]
                                tunnel: 1.0 ("Flowrate(ul/min)") -> [w870 w879 w897 w906 w915 w924]
                                frame #0 {
                                n610 = Index Array(array=w871, index=0) -> (element=w874:dbl)
                                n611 = Greater Than 0?(x=w874) -> (x > 0?=w873:bool)
                                n612 = case shown="True" w873 {
                                tunnel: w872 -> [_ w877]
                                tunnel: w870 -> [_ w876]
                                frame False {
                                }
                                frame True {
                                n613 = call "PumpDispense.vi"("Flowrate(ul/min)"=w876, "Pump Address"="g", "Pump COMM Port"=w877) -> ()  [unwired: 7 in, 2 out]
                                }
                                }
                                }
                                frame #1 {
                                n614 = Index Array(array=w880, index=1) -> (element=w882:dbl)
                                n615 = Greater Than 0?(x=w882) -> (x > 0?=w881:bool)
                                n616 = case shown="False" w881 {
                                tunnel: w879 -> [_ w886]
                                tunnel: w884 -> [_ w885]
                                frame False {
                                }
                                frame True {
                                n617 = local read "Syringe_pump?"() -> (w887:bool)
                                n618 = case shown="False" w887 {
                                tunnel: w886 -> [w888 _]
                                tunnel: w885 -> [w889 _]
                                frame False {
                                n619 = call "PumpDispense.vi"("Flowrate(ul/min)"=w888, "Pump Address"="j", "Pump COMM Port"=w889) -> ()  [unwired: 7 in, 2 out]
                                }
                                frame True {
                                w896 = u16 0 items=["Infuse", "Withdraw"] ("Run Direction (0:Infuse)")
                                w892 = u32 4 items=["milliliters per hour (ml/hr)", "milliliters per minute (ml/min)", "milliliters per second (ml/sec)", "microliters per hour (ul/hr)", "microliters per minute (ul/min)", "microliters per second (ul/sec)", "nanoliters per hour (nl/hr)", "nanoliters per minute (nl/min)", "nanoliters per second (nl/sec)", "picoliters per hour (pl/hr)", "picoliters per minute (pl/min)", "picoliters per second (pl/sec)"] ("Flow Rate Units (1:ml/min)")
                                w893 = u16 0 items=["Infuse", "Withdraw"] ("Pump Direction (0:Infuse)")
                                n620 = local read "COMM Port:: Harvard Syringe Pump"() -> (w894:refnum<visa-resource-name>)
                                n621 = call <instrlib>:"Configure Flow Rate & Direction.vi"("VISA resource name"=w894, "Pump Direction (0:Infuse)"=w893, "Flow Rate (5.00)"=i8 2 ("Pump Address"), "Flow Rate Units (1:ml/min)"=w892) -> ("VISA resource name out"=w895:refnum<visa-resource-name>)  [unwired: 10 in, 1 out]
                                n622 = call <instrlib>:"Start Pump.vi"("Run Direction (0:Infuse)"=w896, "VISA resource name"=w895) -> ()  [unwired: 8 in, 2 out]
                                }
                                }
                                }
                                }
                                }
                                frame #2 {
                                n623 = Index Array(array=w899, index=2) -> (element=w900:dbl)
                                n624 = Greater Than 0?(x=w900) -> (x > 0?=w898:bool)
                                n625 = case shown="True" w898 {
                                tunnel: w902 -> [_ w904]
                                tunnel: w897 -> [_ w903]
                                frame False {
                                }
                                frame True {
                                n626 = call "PumpDispense.vi"("Flowrate(ul/min)"=w903, "Pump Address"="i", "Pump COMM Port"=w904) -> ()  [unwired: 7 in, 2 out]
                                }
                                }
                                }
                                frame #3 {
                                n627 = Index Array(array=w909, index=3) -> (element=w910:dbl)
                                n628 = Greater Than 0?(x=w910) -> (x > 0?=w908:bool)
                                n629 = case shown="True" w908 {
                                tunnel: w907 -> [_ w913]
                                tunnel: w906 -> [_ w912]
                                frame False {
                                }
                                frame True {
                                n630 = call "PumpDispense.vi"("Flowrate(ul/min)"=w912, "Pump Address"="e", "Pump COMM Port"=w913) -> ()  [unwired: 7 in, 2 out]
                                }
                                }
                                }
                                frame #4 {
                                n631 = Index Array(array=w918, index=4) -> (element=w919:dbl)
                                n632 = Greater Than 0?(x=w919) -> (x > 0?=w917:bool)
                                n633 = case shown="True" w917 {
                                tunnel: w916 -> [_ w922]
                                tunnel: w915 -> [_ w921]
                                frame False {
                                }
                                frame True {
                                n634 = call "PumpDispense.vi"("Flowrate(ul/min)"=w921, "Pump Address"="f", "Pump COMM Port"=w922) -> ()  [unwired: 7 in, 2 out]
                                }
                                }
                                }
                                frame #5 {
                                n635 = Index Array(array=w925, index=5) -> (element=w927:dbl)
                                n636 = Greater Than 0?(x=w927) -> (x > 0?=w926:bool)
                                n637 = case shown="True" w926 {
                                tunnel: w929 -> [_ w931]
                                tunnel: w924 -> [_ w930]
                                frame False {
                                }
                                frame True {
                                n638 = call "PumpDispense.vi"("Flowrate(ul/min)"=w930, "Pump Address"="h", "Pump COMM Port"=w931) -> ()  [unwired: 7 in, 2 out]
                                }
                                }
                                }
                                }
                                }
                                frame #1 {
                                n639 = while {
                                stop <- w938 stop-if-true
                                n640 = local read "Phase_Sensor_voltage"() -> (w933:dbl)
                                n641 = script code="organic_phase = 0;\nif start_phase_time \n   start_phase_timer = tic;\n   start_phase_time = 0;\nelse\n  %ignore phase sensor values\n  %if not(phase_sensor_val >2.9 && phase_sensor_val <3.8)\n    %    start_phase_timer = tic;\n   %end\n\n   end_phase_time =  toc(start_phase_timer )\n\n   if end_phase_time > 2\n       organic_phase = 1;\n       start_phase_time = 1;\n   end\n\nend"("phase_sensor_val"=w933) -> ("organic_phase"=w935:dbl)  [unwired: 1 in, 1 out]
                                n642 = local read "Stop"() -> (w937:bool)
                                n643 = Not Equal To 0?(x=w935) -> (x != 0?=w936:bool)
                                n644 = Or(x=w936, y=w937) -> (x .or. y?=w938:bool)
                                n645 = Wait (ms)(milliseconds to wait=u32 300) -> ()  [unwired: 1 out]
                                }
                                }
                                frame #2 {
                                n646 = local read "Stop"() -> (w941:bool)
                                n647 = Not(x=w941) -> (.not. x?=w940:bool)
                                n648 = local read "Sample Valve COMM::Port"() -> (w942:refnum<visa-resource-name>)
                                n649 = case shown="True" w940 {
                                tunnel: w942 -> [_ w944]
                                tunnel: w939 -> [_ w943]
                                frame False {
                                }
                                frame True {
                                n650 = flat-sequence {
                                tunnel: w943 -> [w946]
                                tunnel: w944 -> [w956]
                                frame #0 {
                                n651 = local read "Sample Valve COMM::Port"() -> (w945:refnum<visa-resource-name>)
                                n652 = flat-sequence {
                                tunnel: w948 -> [w953]
                                tunnel: [w953] -> w947
                                frame #0 {
                                n653 = Wait (ms)(milliseconds to wait=u32 500) -> ()  [unwired: 1 out]
                                }
                                }
                                n654 = call-poly <vilib>:"Digital Write.vi"("Output Value"=FALSE, "DO Channel"=u8 22, "LINX Resource"=w947) -> ()  [unwired: 7 in, 2 out]
                                n655 = call-poly <vilib>:"Digital Write.vi"("Output Value"=TRUE, "DO Channel"=u8 22, "LINX Resource"=w946) -> ("LINX Resource"=w948:T10)  [unwired: 7 in, 1 out]
                                n656 = call "NanoValve Inject.vi"("VISA resource name"=w945) -> ()  [unwired: 10 in, 1 out]
                                }
                                frame #1 {
                                n657 = Wait (ms)(milliseconds to wait=u32 2000) -> ()  [unwired: 1 out]
                                }
                                frame #2 {
                                n658 = call "NanoValve Load.vi"("VISA resource name"=w956) -> ()  [unwired: 10 in, 1 out]
                                }
                                }
                                }
                                }
                                }
                                frame #3 {
                                n659 = local read "Stop"() -> (w962:bool)
                                n660 = local read "Bay Parameters"() -> (w958:T2)
                                n661 = Unbundle By Name(w958) -> ("Hplc Wait time(min)"=w960:dbl)
                                n662 = Not(x=w962) -> (.not. x?=w961:bool)
                                n663 = case shown="True" w961 {
                                tunnel: w960 -> [_ w967]
                                tunnel: [errorcluster {"status"=FALSE, "code"=0, "source"=""} ("error out") w966] -> w959
                                tunnel: w958 -> [_ w965]
                                tunnel: w957 -> [_ w964]
                                frame False {
                                }
                                frame True {
                                n664 = flat-sequence {
                                tunnel: w967 -> [w969]
                                tunnel: w964 -> [w978]
                                tunnel: [w989] -> w966
                                tunnel: w965 -> [w988]
                                frame #0 {
                                # "Wait till for HPLC Method"
                                n665 = script code="start = tic;"() -> ("??"=w968:errorcluster)  [unwired: 1 in]
                                n666 = while {
                                tunnel: w969 -> [w971]
                                tunnel: w968 -> [w970]
                                stop <- w977 stop-if-true
                                n667 = Multiply(x=w971, y=60.0) -> (x*y=w972:dbl)
                                n668 = script code="end1 = toc(start);\nflush_time = 0;\nif end1 > hplc_wait_time\n   flush_time = 1;\nend"("??"=w970, "hplc_wait_time"=w972) -> ("flush_time"=w974:dbl)  [unwired: 1 out]
                                n669 = local read "Stop"() -> (w976:bool)
                                n670 = Not Equal To 0?(x=w974) -> (x != 0?=w975:bool)
                                n671 = Or(x=w975, y=w976) -> (x .or. y?=w977:bool)
                                }
                                }
                                frame #1 {
                                n672 = flat-sequence {
                                tunnel: w980 -> [w985]
                                tunnel: [w985] -> w979
                                frame #0 {
                                n673 = Wait (ms)(milliseconds to wait=u32 500) -> ()  [unwired: 1 out]
                                }
                                }
                                n674 = call-poly <vilib>:"Digital Write.vi"("Output Value"=FALSE, "DO Channel"=u8 24, "LINX Resource"=w978) -> ("LINX Resource"=w980:T10)  [unwired: 7 in, 1 out]
                                n675 = call-poly <vilib>:"Digital Write.vi"("Output Value"=TRUE, "DO Channel"=u8 24, "LINX Resource"=w979) -> ()  [unwired: 7 in, 2 out]
                                }
                                frame #2 {
                                n676 = Wait (ms)(milliseconds to wait=u32 30000) -> ()  [unwired: 1 out]
                                }
                                frame #3 {
                                n677 = Unbundle By Name(w988) -> ("hplc File Name"=w990:string)
                                n678 = call "hplc_analyze.vi"("File Path"=w990) -> ("error out"=w989:errorcluster)  [unwired: 10 in]
                                }
                                }
                                }
                                }
                                }
                                frame #4 {
                                n679 = Unbundle By Name(w992) -> ("status"=w993:bool)
                                n680 = case shown="False" w993 {
                                tunnel: w991 -> [_ w994]
                                frame False {
                                }
                                frame True {
                                n681 = while {
                                tunnel: w994 -> [w996]
                                stop <- w995 stop-if-true
                                w1001 = "An error occured while trying to read HPLC data. " ("message")
                                n682 = local write "Error Message"(w1001) -> ()
                                n683 = call <vilib>:"Three Button Dialog.vi"("Right Button Text (\"Cancel\")"="STOP EXPs" ("F button name (\"Cancel\")"), "Center Button Text (\"No\")"="REDO" ("T button name (\"OK\")"), "Left Button Text (\"Yes\")"="REREAD" ("T button name (\"OK\")"), "message"=w1001) -> ("Which Button?"=w997:T19)  [unwired: 7 in]
                                n684 = case shown="\"Left Button\"" w997 {
                                tunnel: w996 -> [_ _ w1008 _]
                                tunnel: [TRUE TRUE w1007 w1010] -> w995
                                frame "Right Button" {
                                w1002 = TRUE ("Setup Error")
                                n685 = local write "System Error"(w1002) -> ()
                                n686 = local write "Setup Error"(w1002) -> ()
                                n687 = script code="system_error = 1"() -> ()  [unwired: 1 in, 1 out]
                                n688 = local write "Stop"(w1002) -> ()
                                }
                                frame "Center Button" {
                                n689 = script code="redo = true;\nopt_ctr = 1;\nCurrExp = CurrExp + 1;\nncall0 = ncall0 +1;\nif req_ctr == req_tot\n       opt_ctr = 3;\n  else\n     req_ctr = req_ctr +1;\nend"() -> ()  [unwired: 1 in, 1 out]
                                }
                                frame "Left Button" {
                                n690 = Unbundle By Name(w1008) -> ("hplc File Name"=w1009:string)
                                n691 = call "hplc_analyze.vi"("File Path"=w1009) -> ("error out"=w1005:errorcluster)  [unwired: 10 in]
                                n692 = Unbundle By Name(w1005) -> ("status"=w1006:bool)
                                n693 = Not(x=w1006) -> (.not. x?=w1007:bool)
                                }
                                frame "Window Close" {
                                w1010 = TRUE
                                n694 = local write "Setup Error"(w1010) -> ()
                                n695 = script code="system_error = 1"() -> ()  [unwired: 1 in, 1 out]
                                n696 = local write "Stop"(w1010) -> ()
                                }
                                }
                                }
                                }
                                }
                                }
                                frame #5 {
                                n697 = disable-structure shown="Disabled" {
                                frame Disabled {
                                n698 = flat-sequence {
                                tunnel: w1012 -> [w1017]
                                tunnel: [w1017] -> w1011
                                frame #0 {
                                n699 = Wait (ms)(milliseconds to wait=u32 500) -> ()  [unwired: 1 out]
                                }
                                }
                                n700 = call-poly <vilib>:"Digital Write.vi"("Output Value"=FALSE, "DO Channel"=u8 22) -> ("LINX Resource"=w1012:T10)  [unwired: 8 in, 1 out]
                                n701 = call-poly <vilib>:"Digital Write.vi"("Output Value"=TRUE, "DO Channel"=u8 22, "LINX Resource"=w1011) -> ()  [unwired: 7 in, 2 out]
                                }
                                frame Enabled {
                                }
                                }
                                }
                                }
                                }
                                }
                              }
                              frame #2 {
                                n702 = script code="C_measured =Conc;\nFvalues(end +1,:) = [Conc];"() -> ()  [unwired: 1 in, 1 out]
                                n703 = local write "HPLC Analysis"(TRUE ("HPLC Analysis")) -> ()
                              }
                            }
                          }
                          frame #4 {
                            n704 = local read "Stop"() -> (w1021:bool)
                            n705 = Not(x=w1021) -> (.not. x?=w1020:bool)
                            n706 = case shown="True" w1020 {
                              tunnel: [1.0 w1032] -> w1022
                              frame False {
                              }
                              frame True {
                                # "Save data to excel file"
                                n707 = local read "Bay Parameters"() -> (w1030:T2)
                                n708 = Unbundle By Name(w1030) -> ("Total Number of Experiments 2"=w1029:dbl)
                                n709 = script code="analyze_labview_results"("ncall"=w1029) -> ("terminate"=w1032:dbl, "ncall0"=w1031:dbl, "experiment_history"=w1027:dbl[][], "Pbest"=w1025:dbl[], "Tbest"=w1026:dbl[], "best_exp_num"=w1024:dbl)  [unwired: 1 in, 1 out]
                                n710 = local write "Flowrates(ul/min)_best"(w1025) -> ()
                                n711 = local write "temperature_best"(w1026) -> ()
                                n712 = local write "best_exp_num"(w1024) -> ()
                                n713 = local write "Current Experiment"(w1031) -> ()
                                n714 = local write "Total Number of Experiments"(w1029) -> ()
                                n715 = call-poly <vilib>:"Array To Matrix.vi"("Real 2D Array"=w1027) -> ("Real Matrix"=w1028:T18)
                                n716 = local write "experiment history"(w1028) -> ()
                              }
                            }
                          }
                          frame #5 {
                            n717 = local read "Num_exp_till_pause"() -> (w1034:i32)
                            n718 = Increment(x=w1034) -> (x+1=w1033:i32)
                            n719 = local write "Num_exp_till_pause"(w1033) -> ()
                          }
                          frame #6 {
                            # "Pause System"
                            n720 = local read "Bay Parameters"() -> (w1042:T2)
                            n721 = Unbundle By Name(w1042) -> ("Num_conditons_per_wait"=w1041:dbl)
                            n722 = local read "Num_exp_till_pause"() -> (w1040:i32)
                            n723 = Equal?(x=w1041, y=w1040) -> (x = y?=w1039:bool)
                            n724 = local read "Run_Stop_cluster"() -> (w1036:T7)
                            n725 = Unbundle By Name(w1036) -> ("Stop Run Button"=w1038:bool)
                            n726 = Or(x=w1038, y=w1039) -> (x .or. y?=w1037:bool)
                            n727 = case shown="True" w1037 {
                              tunnel: w1041 -> [w1045 _]
                              tunnel: w1040 -> [w1046 _]
                              tunnel: w1036 -> [_ w1048]
                              frame False {
                                n728 = Greater?(x=w1046, y=w1045) -> (0:w1044:bool)
                                n729 = case shown="True" w1044 {
                                frame False {
                                }
                                frame True {
                                n730 = local write "Num_exp_till_pause"(0 ("Num_exp_till_pause")) -> ()
                                }
                                }
                              }
                              frame True {
                                n731 = flat-sequence {
                                tunnel: w1048 -> [w1076]
                                frame #0 {
                                w1052 = string[] ["e", "f", "g", "h", "i", "j"]
                                # "Turn off pumps and stop controling temperature"
                                n732 = stacked-sequence {
                                frame #0 {
                                n733 = local write "Temperature Control 1"(FALSE ("Temperature Control 1")) -> ()
                                }
                                frame #1 {
                                n734 = local write "Temperature Control 2"(FALSE ("Temperature Control 2")) -> ()
                                }
                                frame #2 {
                                n735 = local write "Temperature Control 3"(FALSE ("Temperature Control 3")) -> ()
                                }
                                frame #3 {
                                n736 = local write "Temperature Control 4"(FALSE ("Temperature Control 4")) -> ()
                                }
                                frame #4 {
                                n737 = local write "Temperature Control 5"(FALSE ("Temperature Control 5")) -> ()
                                }
                                }
                                n738 = local read "COMM Port:: Harvard Syringe Pump"() -> (w1050:refnum<visa-resource-name>)
                                n739 = local read "Syringe_pump?"() -> (w1049:bool)
                                n740 = local read "COMM Port :: Milligat Pumps"() -> (w1051:refnum<visa-resource-name>)
                                n741 = Array Size(array=w1052) -> (size(s)=w1053:i32)
                                n742 = case shown="True" w1049 {
                                tunnel: w1050 -> [_ w1061]
                                frame False {
                                }
                                frame True {
                                n743 = call <instrlib>:"Stop Pump.vi"("VISA resource name"=w1061) -> ()  [unwired: 9 in, 2 out]
                                }
                                }
                                n744 = for {
                                N: w1053 -> [_]
                                tunnel: w1052 -> [w1059] mode=indexing
                                tunnel: w1051 -> [w1060]
                                n745 = call "PumpStop.vi"("Pump Address"=w1059, "Pump COMM Port"=w1060) -> ()  [unwired: 9 in, 1 out]
                                }
                                }
                                frame #1 {
                                n746 = local read "Stop"() -> (w1064:bool)
                                n747 = Not(x=w1064) -> (.not. x?=w1063:bool)
                                n748 = case shown="True" w1063 {
                                frame False {
                                }
                                frame True {
                                n749 = while {
                                stop <- w1070 stop-if-true
                                # "Wait till user confirms system resume"
                                n750 = Two Button Dialog(message="System is currently paused. Refill Syringes, flush lines, then press OK to continue optimization.\nOr Redo to repeat condition ", 1:"REDO" ("F button name (\"Cancel\")"), 2:"OK" ("Left Button Text (\"Yes\")")) -> (T button?=w1066:bool)
                                n751 = case shown="False" w1066 {
                                tunnel: [TRUE TRUE] -> w1065
                                frame False {
                                n752 = script code="redo = true;"() -> ()  [unwired: 1 in, 1 out]
                                }
                                frame True {
                                }
                                }
                                n753 = local read "Stop"() -> (w1071:bool)
                                n754 = Or(x=w1065, y=w1071) -> (x .or. y?=w1070:bool)
                                }
                                }
                                }
                                n755 = local write "stop_xl_write"(TRUE ("stop_xl_write")) -> ()
                                }
                                frame #2 {
                                n756 = local write "Num_exp_till_pause"(0 ("Num_exp_till_pause")) -> ()
                                n757 = Bundle By Name(cluster=w1076, "Stop Run Button"=FALSE) -> (w1074:T7)
                                n758 = local write "Run_Stop_cluster"(w1074) -> ()
                                }
                                }
                              }
                            }
                          }
                          frame #7 {
                            w1079 = FALSE
                            n759 = local write "Equlibrating Temperature"(w1079) -> ()
                            n760 = local write "Calculate condition"(w1079) -> ()
                            n761 = local write "Flushing System"(w1079) -> ()
                            n762 = local write "HPLC Analysis"(w1079) -> ()
                            n763 = local write "stop_xl_write"(TRUE ("stop_xl_write")) -> ()
                          }
                        }
                        n764 = while {
                          stop <- w1106 stop-if-true
                          n765 = flat-sequence {
                            frame #0 {
                              n766 = script code="save_excel_time_data;"() -> ()  [unwired: 1 in, 1 out]
                            }
                            frame #1 {
                              n767 = Wait (ms)(milliseconds to wait=u32 30000) -> ()  [unwired: 1 out]
                            }
                          }
                          n768 = local read "Stop"() -> (w1107:bool)
                          n769 = local read "stop_xl_write"() -> (w1105:bool)
                          n770 = Or(x=w1105, y=w1107) -> (x .or. y?=w1106:bool)
                        }
                      }
                    }
                  }
                }
                n771 = Greater?(x=w602, y=w603) -> (0:w610:bool)
                n772 = Equal?(x=w608, y=1.0) -> (x = y?=w604:bool)
                n773 = local read "Stop"() -> (w611:bool)
                n774 = Or(x=w611, y=w610) -> (x .or. y?=w607:bool)
                n775 = Or(x=w604, y=w607) -> (x .or. y?=w606:bool)
                n776 = case shown="True" w604 {
                  frame False {
                  }
                  frame True {
                    w615 = u16 2 items=["System  Error", "System Running", "System Standby"] ("System Status")
                    n777 = local write "Stop"(TRUE ("Stop")) -> ()
                    n778 = local write "System Status"(w615) -> ()
                  }
                }
                "Optimization_loop_index" <- w612
              }
            }
          }
          n779 = while {
            tunnel: w590 -> [w1202]
            stop <- w1205 stop-if-true
            n780 = local read "Temperature Control 3"() -> (w1203:bool)
            n781 = local read "running?"() -> (w1201:bool)
            n782 = And(x=w1201, y=w1203) -> (x .and. y?=w1204:bool)
            n783 = case shown="True" w1204 {
              tunnel: w1202 -> [_ w1208]
              frame False {
                n784 = local write "Temp SS? 3"(TRUE) -> ()
              }
              frame True {
                # "Bay 3 Temperature Controller"
                n785 = local read "Temperature SP 3"() -> (w1209:dbl)
                n786 = local read "Temperature 3"() -> (w1212:dbl)
                n787 = Subtract(x=w1212, y=w1209) -> (x-y=w1221:dbl)
                n788 = Absolute Value(x=w1221) -> (abs(x)=w1223:dbl)
                n789 = Less Or Equal?(x=w1223, y=1.2) -> (x <= y?=w1220:bool)
                n790 = local write "Temp SS? 3"(w1220) -> ()
                n791 = local read "SSR Duration 3"() -> (w1230:dbl)
                n792 = call-poly <vilib>:"PID Online Autotuning.vi"("setpoint"=w1209, "manipulated variable"=w1230, "autotuning parameters"=T9 {"type of controller"=enum."PID", "relay cycles"=3, "relay amplitude"=1.0, "control specifications"=enum."Normal", "PV noise level"=0.1} ("Autotuning Parameters R1"), "process variable"=w1212, "PID gains in"=T8 {"Proportional gain Kc"=0.38538, "Integral time Ti (sec)"=0.524375, "Derivative time Ti (sec)"=0.12585} ("PID gains 2")) -> ("setpoint out"=w1228:dbl, "process variable out"=w1229:dbl, "PID gains out"=w1232:T17)  [unwired: 6 in, 2 out]
                n793 = Greater?(x=w1209, y=w1212) -> (0:w1219:bool)
                n794 = call <vilib>:"PID Autotuning (Temperature).vi"("desired temperature"=w1228, "measured temperature"=w1229, "PID gains in"=w1232, "output range"=cluster{"output high":dbl, "output low":dbl} {"output high"=3.0, "output low"=-1.0} ("Output range")) -> ("output"=w1225:dbl)  [unwired: 12 in, 3 out]
                n795 = Multiply(x=1000.0, y=w1225) -> (x*y=w1227:dbl)
                n796 = local write "SSR Duration 3"(w1225) -> ()
                n797 = Greater Than 0?(x=w1227) -> (x > 0?=w1218:bool)
                n798 = And(x=w1218, y=w1219) -> (x .and. y?=w1216:bool)
                n799 = Subtract(x=w1212, y=10.0) -> (x-y=w1214:dbl)
                n800 = Less?(x=w1214, y=w1209) -> (x < y?=w1217:bool)
                n801 = And(x=w1217, y=w1216) -> (x .and. y?=w1215:bool)
                n802 = case shown="True" w1215 {
                  tunnel: [errorcluster {"status"=FALSE, "code"=0, "source"=""} ("error out") w1244] -> _
                  tunnel: 4 -> [_ w1242]
                  tunnel: w1227 -> [w1238 w1243]
                  tunnel: [0.0 w1246] -> w1210
                  tunnel: w1209 -> [_ w1245]
                  tunnel: w1208 -> [_ w1241]
                  frame False {
                    n803 = Absolute Value(x=w1238) -> (abs(x)=w1239:dbl)
                    n804 = Wait (ms)(milliseconds to wait=w1239) -> ()  [unwired: 1 out]
                  }
                  frame True {
                    n805 = call "TurnOnRelayArduino.vi"("channel"=w1242, "duration"=w1243, "LINX Resource"=w1241) -> ("error out"=w1244:errorcluster)  [unwired: 7 in, 1 out]
                    n806 = script code="tempdiff3= SP3 - T3;\nif tempdiff3 > 10\n  if slope3 < .01\n     temp_check3 = temp_check3 + 1;\n  else\n      temp_check3 =0;\n  end\nend\n\nif temp_check3 > 9\n  temp_error3 = 1\nend"("SP3"=w1245) -> ("temp_error3"=w1246:dbl)  [unwired: 1 in, 1 out]
                  }
                }
                n807 = Not Equal To 0?(x=w1210) -> (x != 0?=w1211:bool)
                n808 = case shown="True" w1211 {
                  frame False {
                  }
                  frame True {
                    n809 = local write "Error Message"("Bay 3 Temperature Heating Error") -> ()
                  }
                }
                n810 = case shown="True" w1211 {
                  tunnel: w1211 -> [_ w1236]
                  frame False {
                  }
                  frame True {
                    n811 = local write "System Error"(w1236) -> ()
                    n812 = local write "Stop"(w1236) -> ()
                  }
                }
              }
            }
            n813 = Wait (ms)(milliseconds to wait=u32 400) -> ()  [unwired: 1 out]
            n814 = local read "Stop"() -> (w1205:bool)
          }
          n815 = while {
            tunnel: w590 -> [w1156]
            stop <- w1159 stop-if-true
            n816 = local read "running?"() -> (w1155:bool)
            n817 = Wait (ms)(milliseconds to wait=u32 400) -> ()  [unwired: 1 out]
            n818 = local read "Temperature Control 4"() -> (w1158:bool)
            n819 = And(x=w1155, y=w1158) -> (x .and. y?=w1157:bool)
            n820 = case shown="True" w1157 {
              tunnel: w1156 -> [_ w1162]
              frame False {
                n821 = local write "Temp SS? 4"(TRUE ("Temp SS? 4")) -> ()
              }
              frame True {
                # "Bay 4 Temperature Controller"
                n822 = local read "Temperature SP 4"() -> (w1165:dbl)
                n823 = local read "Temperature 4"() -> (w1168:dbl)
                n824 = Subtract(x=w1168, y=w1165) -> (x-y=w1175:dbl)
                n825 = Absolute Value(x=w1175) -> (abs(x)=w1177:dbl)
                n826 = Less Or Equal?(x=w1177, y=1.2) -> (x <= y?=w1174:bool)
                n827 = local write "Temp SS? 4"(w1174) -> ()
                n828 = local read "SSR Duration 4"() -> (w1178:dbl)
                n829 = call-poly <vilib>:"PID Online Autotuning.vi"("setpoint"=w1165, "manipulated variable"=w1178, "autotuning parameters"=T9 {"type of controller"=enum."PID", "relay cycles"=3, "relay amplitude"=1.0, "control specifications"=enum."Normal", "PV noise level"=0.1} ("Autotuning Parameters R1"), "process variable"=w1168, "PID gains in"=T8 {"Proportional gain Kc"=0.38538, "Integral time Ti (sec)"=0.524375, "Derivative time Ti (sec)"=0.12585} ("PID gains 2")) -> ("setpoint out"=w1180:dbl, "process variable out"=w1181:dbl, "PID gains out"=w1183:T17)  [unwired: 6 in, 2 out]
                n830 = call <vilib>:"PID Autotuning (Temperature).vi"("desired temperature"=w1180, "measured temperature"=w1181, "PID gains in"=w1183, "output range"=cluster{"output high":dbl, "output low":dbl} {"output high"=3.0, "output low"=-1.0} ("Output range")) -> ("output"=w1179:dbl)  [unwired: 12 in, 3 out]
                n831 = Subtract(x=w1168, y=10.0) -> (x-y=w1167:dbl)
                n832 = Less?(x=w1167, y=w1165) -> (x < y?=w1169:bool)
                n833 = Multiply(x=1000.0, y=w1179) -> (x*y=w1187:dbl)
                n834 = Greater?(x=w1165, y=w1168) -> (0:w1173:bool)
                n835 = Greater Than 0?(x=w1187) -> (x > 0?=w1172:bool)
                n836 = local write "SSR Duration 4"(w1179) -> ()
                n837 = And(x=w1172, y=w1173) -> (x .and. y?=w1171:bool)
                n838 = And(x=w1169, y=w1171) -> (x .and. y?=w1170:bool)
                n839 = case shown="True" w1170 {
                  tunnel: [errorcluster {"status"=FALSE, "code"=0, "source"=""} ("error out") w1198] -> _
                  tunnel: 5 -> [_ w1196]
                  tunnel: w1187 -> [w1192 w1197]
                  tunnel: w1165 -> [_ w1200]
                  tunnel: [0.0 w1199] -> w1164
                  tunnel: w1162 -> [_ w1195]
                  frame False {
                    n840 = Absolute Value(x=w1192) -> (abs(x)=w1193:dbl)
                    n841 = Wait (ms)(milliseconds to wait=w1193) -> ()  [unwired: 1 out]
                  }
                  frame True {
                    n842 = call "TurnOnRelayArduino.vi"("channel"=w1196, "duration"=w1197, "LINX Resource"=w1195) -> ("error out"=w1198:errorcluster)  [unwired: 7 in, 1 out]
                    n843 = script code="tempdiff4= SP4 - T4;\nif tempdiff4 > 10\n  if slope4 < .01\n     temp_check4 = temp_check4 + 1;\n  else\n      temp_check4 =0;\n  end\nend\n\nif temp_check4 > 9\n  temp_error4 = 1\nend"("SP4"=w1200) -> ("temp_error4"=w1199:dbl)  [unwired: 1 in, 1 out]
                  }
                }
                n844 = Not Equal To 0?(x=w1164) -> (x != 0?=w1163:bool)
                n845 = case shown="True" w1163 {
                  frame False {
                  }
                  frame True {
                    n846 = local write "Error Message"("Bay 4 Temperature Heating Error") -> ()
                  }
                }
                n847 = case shown="True" w1163 {
                  tunnel: w1163 -> [_ w1190]
                  frame False {
                  }
                  frame True {
                    n848 = local write "System Error"(w1190) -> ()
                    n849 = local write "Stop"(w1190) -> ()
                  }
                }
              }
            }
            n850 = local read "Stop"() -> (w1159:bool)
          }
          n851 = while {
            stop <- w595 stop-if-true
            n852 = script code="TempArr1=circshift(TempArr1,9);\nTempArr2=circshift(TempArr2,9);\nTempArr3=circshift(TempArr3,9);\nTempArr4=circshift(TempArr4,9);\nTempArr5=circshift(TempArr5,9);\n\nTempArr1(10)=T1;\nTempArr2(10)=T2;\nTempArr3(10)=T3;\nTempArr4(10)=T4;\nTempArr5(10)=T5;\n\n[slope1 temp] = polyfit([1,2,3,4,5,6,7,8,9,10]',TempArr1,1);\nslope1 = slope1(1);\n[slope2 temp] = polyfit([1,2,3,4,5,6,7,8,9,10]',TempArr2,1);\nslope2= slope2(1);\n[slope3 temp] = polyfit([1,2,3,4,5,6,7,8,9,10]',TempArr3,1);\nslope3 = slope3(1);\n[slope4 temp] = polyfit([1,2,3,4,5,6,7,8,9,10]',TempArr4,1);\nslope4 = slope4(1);\n[slope5 temp] = polyfit([1,2,3,4,5,6,7,8,9,10]',TempArr5,1);\nslope5 = slope5(1);"() -> ()  [unwired: 1 in, 1 out]
            n853 = Wait (ms)(milliseconds to wait=u32 600) -> ()  [unwired: 1 out]
            n854 = local read "Stop"() -> (w595:bool)
          }
          n855 = while {
            tunnel: w590 -> [w1110]
            stop <- w1113 stop-if-true
            n856 = local read "running?"() -> (w1109:bool)
            n857 = local read "Temperature Control 5"() -> (w1111:bool)
            n858 = And(x=w1109, y=w1111) -> (x .and. y?=w1112:bool)
            n859 = case shown="True" w1112 {
              tunnel: w1110 -> [_ w1116]
              frame False {
                n860 = local write "Temp SS? 5"(TRUE ("Temp SS? 5")) -> ()
              }
              frame True {
                # "Bay 5 Temperature Controller"
                n861 = local read "SSR Duration 5"() -> (w1132:dbl)
                n862 = local read "Temperature SP 5"() -> (w1118:dbl)
                n863 = local read "Temperature 5"() -> (w1121:dbl)
                n864 = Subtract(x=w1121, y=w1118) -> (x-y=w1129:dbl)
                n865 = Absolute Value(x=w1129) -> (abs(x)=w1131:dbl)
                n866 = Less Or Equal?(x=w1131, y=1.2) -> (x <= y?=w1128:bool)
                n867 = local write "Temp SS? 5"(w1128) -> ()
                n868 = call-poly <vilib>:"PID Online Autotuning.vi"("setpoint"=w1118, "manipulated variable"=w1132, "autotuning parameters"=T9 {"type of controller"=enum."PID", "relay cycles"=3, "relay amplitude"=1.0, "control specifications"=enum."Normal", "PV noise level"=0.1} ("Autotuning Parameters R1"), "process variable"=w1121, "PID gains in"=T8 {"Proportional gain Kc"=0.38538, "Integral time Ti (sec)"=0.524375, "Derivative time Ti (sec)"=0.12585} ("PID gains 2")) -> ("setpoint out"=w1134:dbl, "process variable out"=w1135:dbl, "PID gains out"=w1137:T17)  [unwired: 6 in, 2 out]
                n869 = call <vilib>:"PID Autotuning (Temperature).vi"("desired temperature"=w1134, "measured temperature"=w1135, "PID gains in"=w1137, "output range"=cluster{"output high":dbl, "output low":dbl} {"output high"=3.0, "output low"=-1.0} ("Output range")) -> ("output"=w1133:dbl)  [unwired: 12 in, 3 out]
                n870 = Multiply(x=1000.0, y=w1133) -> (x*y=w1141:dbl)
                n871 = Greater?(x=w1118, y=w1121) -> (0:w1126:bool)
                n872 = Greater Than 0?(x=w1141) -> (x > 0?=w1127:bool)
                n873 = local write "SSR Duration 5"(w1133) -> ()
                n874 = And(x=w1127, y=w1126) -> (x .and. y?=w1124:bool)
                n875 = Subtract(x=w1121, y=10.0) -> (x-y=w1122:dbl)
                n876 = Greater?(x=w1122, y=w1118) -> (0:w1125:bool)
                n877 = And(x=w1125, y=w1124) -> (x .and. y?=w1123:bool)
                n878 = case shown="True" w1123 {
                  tunnel: [errorcluster {"status"=FALSE, "code"=0, "source"=""} ("error out") w1152] -> _
                  tunnel: 6 -> [_ w1149]
                  tunnel: w1141 -> [w1146 w1150]
                  tunnel: [0.0 w1154] -> w1119
                  tunnel: w1118 -> [_ w1153]
                  tunnel: w1116 -> [_ w1151]
                  frame False {
                    n879 = Absolute Value(x=w1146) -> (abs(x)=w1147:dbl)
                    n880 = Wait (ms)(milliseconds to wait=w1147) -> ()  [unwired: 1 out]
                  }
                  frame True {
                    n881 = call "TurnOnRelayArduino.vi"("channel"=w1149, "duration"=w1150, "LINX Resource"=w1151) -> ("error out"=w1152:errorcluster)  [unwired: 7 in, 1 out]
                    n882 = script code="tempdiff5= SP5 - T5;\n\nif tempdiff5 > 10\n  if slope5 < .01\n     temp_check5 = temp_check5 + 1;\n  else\n      temp_check5 =0;\n  end\nend\n\nif temp_check5 >9\n  temp_error5 = 1\nend"("SP5"=w1153) -> ("temp_error5"=w1154:dbl)  [unwired: 1 in, 1 out]
                  }
                }
                n883 = Not Equal To 0?(x=w1119) -> (x != 0?=w1117:bool)
                n884 = case shown="True" w1117 {
                  frame False {
                  }
                  frame True {
                    n885 = local write "Error Message"("Bay 5 Temperature Heating Error") -> ()
                  }
                }
                n886 = case shown="True" w1117 {
                  tunnel: w1117 -> [_ w1144]
                  frame False {
                  }
                  frame True {
                    n887 = local write "Stop"(w1144) -> ()
                    n888 = local write "System Error"(w1144) -> ()
                  }
                }
              }
            }
            n889 = Wait (ms)(milliseconds to wait=u32 400) -> ()  [unwired: 1 out]
            n890 = local read "Stop"() -> (w1113:bool)
          }
        }
      }
      n891 = local read "IR Sensor Device"() -> (w62:T6)
      n892 = while {
        tunnel: errorcluster {"status"=FALSE, "code"=0, "source"=""} ("error out") -> [w133]
        tunnel: w62 -> [w152]
        stop <- w173 stop-if-true
        w130 = u8 7 items=["RAM IR raw  Ch1"=4, "RAM IR raw  Ch2"=5, "RAM T_A"=6, "RAM T_OBJ1"=7, "RAM T_OBJ2"=8, "EEPROM_To_max"=32, "EEPROM_To_min"=33, "EEPROM_PWM_CTRL"=34, "EEPROM_Ta_range"=35, "EEPROM_Emissivity_CorrCoeff"=36, "EEPROM_SMBus Address"=46, "EEPROM_ConfigReg"=37] ("Melexis_Cmmds")
        # "Bay 5 Temperature Read"
        # "Bay 4 Temperature Read"
        # "Bay 3 Temperature Read"
        # "Bay 2 Temperature Read"
        # "Bay 1 Temperature Read"
        n893 = local read "Stop"() -> (w173:bool)
        n894 = call "IRSensorNIRead.vi"("error in (no error)"=w133, "Melexis_Cmmds"=w130, "Address"=u8 1, "device reference"=w152) -> ("error out"=w155:errorcluster, "Temperature"=w153:dbl, "device reference out"=w151:T6)  [unwired: 5 in]
        n895 = local write "error out"(w155) -> ()
        n896 = Unbundle By Name(w155) -> ("status"=w154:bool)
        n897 = call-poly <vilib>:"PID Control Input Filter.vi"("input"=w153) -> ("output"=w166:dbl)  [unwired: 4 in]
        n898 = case shown="False" w154 {
          tunnel: w165 -> [w182 _]
          tunnel: [w182 w183] -> w170
          frame False {
            n899 = local write "Temperature 1"(w182) -> ()
          }
          frame True {
            n900 = local read "Temperature 1"() -> (w183:dbl)
          }
        }
        n901 = flat-sequence {
          tunnel: w166 -> [w196]
          tunnel: [w196] -> w165
          tunnel: w151 -> [w195]
          tunnel: [w195] -> w150
          frame #0 {
            n902 = Wait (ms)(milliseconds to wait=u32 100) -> ()  [unwired: 1 out]
          }
        }
        n903 = call "IRSensorNIRead.vi"("error in (no error)"=w133, "Melexis_Cmmds"=w130, "Address"=u8 2, "device reference"=w150) -> ("error out"=w142:errorcluster, "Temperature"=w143:dbl, "device reference out"=w145:T6)  [unwired: 5 in]
        n904 = local write "error out"(w142) -> ()
        n905 = Unbundle By Name(w142) -> ("status"=w147:bool)
        n906 = call-poly <vilib>:"PID Control Input Filter.vi"("input"=w143) -> ("output"=w164:dbl)  [unwired: 4 in]
        n907 = case shown="True" w147 {
          tunnel: w163 -> [w180 _]
          tunnel: [w180 w181] -> w169
          frame False {
            n908 = local write "Temperature 2"(w180) -> ()
          }
          frame True {
            n909 = local read "Temperature 2"() -> (w181:dbl)
          }
        }
        n910 = flat-sequence {
          tunnel: w164 -> [w193]
          tunnel: [w193] -> w163
          tunnel: w145 -> [w192]
          tunnel: [w192] -> w144
          frame #0 {
            n911 = Wait (ms)(milliseconds to wait=u32 100) -> ()  [unwired: 1 out]
          }
        }
        n912 = call "IRSensorNIRead.vi"("error in (no error)"=w133, "Melexis_Cmmds"=w130, "Address"=u8 3, "device reference"=w144) -> ("error out"=w135:errorcluster, "Temperature"=w141:dbl, "device reference out"=w140:T6)  [unwired: 5 in]
        n913 = local write "error out"(w135) -> ()
        n914 = Unbundle By Name(w135) -> ("status"=w136:bool)
        n915 = case shown="False" w136 {
          tunnel: w160 -> [w178 _]
          tunnel: [w178 w179] -> w162
          frame False {
            n916 = local write "Temperature 3"(w178) -> ()
          }
          frame True {
            n917 = local read "Temperature 3"() -> (w179:dbl)
          }
        }
        n918 = call-poly <vilib>:"PID Control Input Filter.vi"("input"=w141) -> ("output"=w161:dbl)  [unwired: 4 in]
        n919 = flat-sequence {
          tunnel: w161 -> [w190]
          tunnel: [w190] -> w160
          tunnel: w140 -> [w189]
          tunnel: [w189] -> w138
          frame #0 {
            n920 = Wait (ms)(milliseconds to wait=u32 100) -> ()  [unwired: 1 out]
          }
        }
        n921 = call "IRSensorNIRead.vi"("error in (no error)"=w133, "Melexis_Cmmds"=w130, "Address"=u8 4, "device reference"=w138) -> ("error out"=w125:errorcluster, "Temperature"=w137:dbl, "device reference out"=w132:T6)  [unwired: 5 in]
        n922 = local write "error out"(w125) -> ()
        n923 = Unbundle By Name(w125) -> ("status"=w127:bool)
        n924 = case shown="True" w127 {
          tunnel: w158 -> [w176 _]
          tunnel: [w176 w177] -> w168
          frame False {
            n925 = local write "Temperature 4"(w176) -> ()
          }
          frame True {
            n926 = local read "Temperature 4"() -> (w177:dbl)
          }
        }
        n927 = call-poly <vilib>:"PID Control Input Filter.vi"("input"=w137) -> ("output"=w159:dbl)  [unwired: 4 in]
        n928 = flat-sequence {
          tunnel: w159 -> [w187]
          tunnel: [w187] -> w158
          tunnel: w132 -> [w186]
          tunnel: [w186] -> w131
          frame #0 {
            n929 = Wait (ms)(milliseconds to wait=u32 100) -> ()  [unwired: 1 out]
          }
        }
        n930 = call "IRSensorNIRead.vi"("error in (no error)"=w133, "Melexis_Cmmds"=w130, "Address"=u8 5, "device reference"=w131) -> ("error out"=w128:errorcluster, "Temperature"=w129:dbl)  [unwired: 5 in, 1 out]
        n931 = local write "error out"(w128) -> ()
        n932 = flat-sequence {
          tunnel: w157 -> [w184]
          tunnel: [w184] -> w156
          frame #0 {
            n933 = Wait (ms)(milliseconds to wait=u32 100) -> ()  [unwired: 1 out]
          }
        }
        n934 = Unbundle By Name(w128) -> ("status"=w126:bool)
        n935 = call-poly <vilib>:"PID Control Input Filter.vi"("input"=w129) -> ("output"=w157:dbl)  [unwired: 4 in]
        n936 = local write "error out"(w133) -> ()
        n937 = Build Array(w170, w169, w162, w168, w156) -> (w172:dbl[])
        n938 = Array To Cluster(array=w172) -> (cluster=→"Teperature Chart":T3)
        n939 = case shown="False" w126 {
          tunnel: w156 -> [w174 _]
          tunnel: [w174 w175] -> w167
          frame False {
            n940 = local write "Temperature 5"(w174) -> ()
          }
          frame True {
            n941 = local read "Temperature 5"() -> (w175:dbl)
          }
        }
        n942 = script code="MATLAB script"("T1"=w170, "T2"=w169, "T3"=w162, "T4"=w168, "T5"=w167) -> ()  [unwired: 1 in, 1 out]
      }
      n943 = while {
        stop <- w88 stop-if-true
        n944 = local read "Pump setpoint(ul/min) 1"() -> (w91:dbl)
        n945 = local read "Pump setpoint(ul/min) 2"() -> (w87:dbl)
        n946 = local read "Pump setpoint(ul/min) 3"() -> (w86:dbl)
        n947 = local read "Pump setpoint(ul/min) 4"() -> (w85:dbl)
        n948 = local read "Pump setpoint(ul/min) 5"() -> (w84:dbl)
        n949 = local read "Pump setpoint(ul/min) 6"() -> (w83:dbl)
        n950 = Build Array(w91, w87, w86, w85, w84, w83) -> (w92:dbl[])
        n951 = Array To Cluster(array=w92) -> (cluster=→"Pump Setpoints Chart":T3)
        n952 = Wait (ms)(milliseconds to wait=u32 5000) -> ()  [unwired: 1 out]
        n953 = local read "Stop"() -> (w88:bool)
      }
      n954 = while {
        stop <- w70 stop-if-true
        n955 = local read "System Error"() -> (w69:bool)
        n956 = Wait (ms)(milliseconds to wait=u32 300) -> ()  [unwired: 1 out]
        n957 = case shown="True" w69 {
          tunnel: [w74 w75] -> w67
          frame False {
            w71 = u16 2 items=["System  Error", "System Running", "System Standby"] ("System Status")
            w72 = u16 1 items=["System  Error", "System Running", "System Standby"] ("System Status")
            n958 = local read "running?"() -> (w73:bool)
            n959 = Select(t=w72, s=w73, f=w71) -> (s? t:f=w74:u16)
          }
          frame True {
            w75 = u16 0 items=["System  Error", "System Running", "System Standby"] ("System Status")
          }
        }
        n960 = local read "Stop"() -> (w70:bool)
        n961 = local write "System Status"(w67) -> ()
      }
      n962 = while {
        tunnel: w61 -> [w76]
        stop <- w82 stop-if-true
        n963 = call-poly <vilib>:"Analog Read.vi"("Analog Channel"=u8 0, "LINX Resource"=w76) -> ("Voltage"=w77:dbl)  [unwired: 6 in, 3 out]
        "Phase_Sensor_voltage" <- w77
        n964 = Wait (ms)(milliseconds to wait=u32 300) -> ()  [unwired: 1 out]
        n965 = Build Array(w77) -> (w79:dbl[])
        n966 = Array To Cluster(array=w79) -> (cluster=→"Phase Sensor Chart":T3)
        n967 = local read "Stop"() -> (w82:bool)
      }
      n968 = while {
        tunnel: w61 -> [w95]
        stop <- w120 stop-if-true
        w102 = 270
        w96 = 600
        w97 = 600
        # "Read Pressure and Flowrate"
        n969 = local read "Stop"() -> (w120:bool)
        n970 = call-poly <vilib>:"Analog Read.vi"("AI Channel(s)"=i32[] [14, 15, 14, 15], "LINX Resource"=w95) -> ("Voltages"=w93:dbl[])  [unwired: 6 in, 3 out]
        n971 = Index Array(array=w93, index=1) -> (element=w116:dbl)
        n972 = Index Array(array=w93, index=0) -> (element=w117:dbl)
        n973 = call-poly <vilib>:"PID Control Input Filter.vi"("input"=w116) -> ("output"=w109:dbl)  [unwired: 4 in]
        n974 = call-poly <vilib>:"PID Control Input Filter.vi"("input"=w117) -> ("output"=w108:dbl)  [unwired: 4 in]
        n975 = Multiply(x=104.96 ("y"), y=w109) -> (x*y=w110:dbl)
        n976 = Multiply(x=104.96 ("y"), y=w108) -> (x*y=w113:dbl)
        n977 = Subtract(x=w110, y=24.077) -> (x-y=w100:dbl)
        n978 = Subtract(x=w113, y=24.077) -> (x-y=w101:dbl)
        n979 = Build Array(w97, w96) -> (w105:i32[])
        n980 = Array To Cluster(array=w105) -> (cluster=→"Flowrate Chart":T4)
        n981 = Build Array(w101, w100) -> (w106:dbl[])
        n982 = local write "Flowrate Sensor 1"(w97) -> ()
        n983 = local write "Flowrate Sensor 2"(w96) -> ()
        n984 = local write "Pressure 1"(w101) -> ()
        n985 = local write "Pressure 2"(w100) -> ()
        n986 = Array To Cluster(array=w106) -> (cluster=→"Pressure Chart":T3)
        n987 = Wait (ms)(milliseconds to wait=u32 500) -> ()  [unwired: 1 out]
        n988 = script code="MATLAB script"("F1"=w97, "F2"=w96, "Pres1"=w101, "Pres2"=w100) -> ()  [unwired: 1 in, 1 out]
        n989 = Greater?(x=w100, y=w102) -> (0:w98:bool)
        n990 = Greater?(x=w101, y=w102) -> (0:w99:bool)
        n991 = case shown="True" w99 {
          frame False {
          }
          frame True {
            w124 = TRUE ("Stop")
            n992 = local write "System Error"(w124) -> ()
            n993 = local write "Stop"(w124) -> ()
            n994 = local write "Error Message"("Pressure Sensor 1 readings above 250psi") -> ()
            n995 = script code="system_error = 1;"() -> ()  [unwired: 1 in, 1 out]
          }
        }
        n996 = case shown="False" w98 {
          frame False {
          }
          frame True {
            w122 = TRUE ("Stop")
            n997 = local write "System Error"(w122) -> ()
            n998 = local write "Error Message"("Pressure Sensor 2 readings above 250psi") -> ()
            n999 = local write "Stop"(w122) -> ()
            n1000 = script code="system_error = 1;"() -> ()  [unwired: 1 in, 1 out]
          }
        }
      }
    }
    frame #3 {
      # "Save and close xml and excel file"
      n1001 = script code="if exist('xl_file','var') & exist('xlApp','var')\n  xlWorkbook.SaveAs(xl_file);\n  xlWorkbook.Close;\n  xlApp.Quit;\n  xlApp.delete;\nend"() -> ()  [unwired: 1 in, 1 out]
    }
    frame #4 {
      w1350 = string[] ["e", "f", "g", "h", "i", "j"]
      # "End communication to hardware"
      n1002 = local read "Syringe_pump?"() -> (w1348:bool)
      n1003 = local read "COMM Port:: Harvard Syringe Pump"() -> (w1349:refnum<visa-resource-name>)
      n1004 = local read "IR Sensor Device"() -> (w1347:T6)
      n1005 = local read "COMM Port :: Milligat Pumps"() -> (w1352:refnum<visa-resource-name>)
      n1006 = call <vilib>:"Close.vi"("LINX Resource"=w1346) -> ()  [unwired: 10 in, 1 out]
      n1007 = Array Size(array=w1350) -> (size(s)=w1351:i32)
      n1008 = case shown="True" w1348 {
        tunnel: w1349 -> [_ w1353]
        frame False {
        }
        frame True {
          n1009 = call <instrlib>:"Stop Pump.vi"("VISA resource name"=w1353) -> ()  [unwired: 9 in, 2 out]
        }
      }
      n1010 = for {
        N: w1351 -> [_]
        tunnel: w1350 -> [w1354] mode=indexing
        tunnel: w1352 -> [w1355]
        n1011 = call "PumpStop.vi"("Pump Address"=w1354, "Pump COMM Port"=w1355) -> ()  [unwired: 9 in, 1 out]
        n1012 = Wait (ms)(milliseconds to wait=u32 100) -> ()  [unwired: 1 out]
      }
      n1013 = call-poly <vilib>:"NI-845x Close Reference.vi"("device reference"=w1347) -> ()  [unwired: 10 in, 1 out]
    }
    frame #5 {
      # "Display Error Messages if necessary"
      n1014 = local read "Error Message"() -> (w1357:string)
      n1015 = One Button Dialog(message=w1357) -> ()  [unwired: 1 in, 1 out]
    }
  }
